vi "WVDIAL_2_OphirPM_v2.3_temp_tune.vi"() -> ()   [LabVIEW 2012]
uses:
  <vilib>/DAQmx/write.llb/DAQmx Write (Digital 1D Bool NChan 1Samp 1Line).vi
  <vilib>/DAQmx/miscellaneous.llb/DAQmx Fill In Error Info.vi
  under_development/AMCS_Data.vi
  <vilib>/Analysis/baseanly.llb/Mean (DBL).vi
  H2O_DIAL/LabVIEW-2012/Scalar_Data.vi
  H2O_DIAL/LabVIEW-2012/Bristol WM V2_31b/CLDevIFace.dll
  <vilib>/Analysis/NI_AALBase.lvlib
panel:
  out "error out 4":errorcluster
  out "error out 3":errorcluster
  out "error out 2":errorcluster
  out "error out":errorcluster
  out "AMCS_Profile":i32=208217
  out "FileHour":i32=17
  out "L_Count":i32=201042
  out "sigma_off_total":dbl[](array[numeric])=[5.545387503084242e-25, 5.506921512625635e-25, 5.468655063160739e-25, 5.430588031815433e-25, 5.39272028507623e-25, 5.35505167878492e-25, 5.317582058036299e-25, 5.280311257273803e-25, 5.243239100182651e-25, 5.206365399736143e-25, 5.169689958185842e-25, 5.133212567065494e-25, 5.096933007194568e-25, 5.060851048742239e-25, 5.024966451178001e-25, 4.989278963386338e-25, 4.953788323632695e-25, 4.918494259626275e-25, 4.883396488574925e-25, 4.848494717236001e-25, 4.813788641946174e-25, 4.779277948683017e-25, 4.744962313158126e-25, 4.710841400843162e-25, 4.676914867043271e-25, 4.643182356986159e-25, 4.609643505899978e-25, 4.576297939040525e-25, 4.543145271851358e-25, 4.510185109959037e-25, 4.477417049336712e-25, 4.444840676323304e-25, 4.412455567763804e-25, 4.3802612910682375e-25, 4.348257404317652e-25, 4.316443456338351e-25, 4.284818986840961e-25, 4.253383526463104e-25, 4.222136596891092e-25, 4.191077710978466e-25, 4.160206372783186e-25, 4.1295220777418144e-25, 4.09902431272516e-25, 4.0687125561240014e-25, 4.038586277999945e-25, 4.0086449401468787e-25, 3.978887996201128e-25, 3.9493148917382813e-25, 3.9199250643855913e-25, 3.890717943910424e-25, 3.8616929523256806e-25, 3.832849503983646e-25, 3.804187005685776e-25, 3.775704856767893e-25, 3.7474024492078913e-25, 3.7192791677202016e-25, 3.691334389844544e-25, 3.6635674860611747e-25, 3.6359778198783013e-25, 3.608564747899254e-25, 3.5813276199740633e-25, 3.5542657792324006e-25, 3.5273785622244977e-25, 3.5006652989779304e-25, 3.474125313105615e-25, 3.447757921904358e-25, 3.421562436422067e-25, 3.3955381615686624e-25, 3.3696843961848715e-25, 3.3440004331667853e-25, 3.318485559484839e-25, 3.2931390563522844e-25, 3.2679601992567473e-25, 3.2429482580501904e-25, 3.218102497081505e-25, 3.1934221752128248e-25, 3.1689065459536094e-25, 3.144554857534307e-25, 3.1203663529904646e-25, 3.096340270240214e-25, 3.072475842173334e-25, 3.0487722967580223e-25, 3.0252288570892426e-25, 3.0018447414936605e-25, 2.9786191636379327e-25, 2.955551332584365e-25, 2.93264045288151e-25, 2.9098857246799783e-25, 2.8872863437846284e-25, 2.8648415018058536e-25, 2.8425503861601494e-25, 2.8204121802703507e-25, 2.798426063570431e-25, 2.7765912116729236e-25, 2.7549067964110224e-25, 2.7333719859787194e-25, 2.711985945027861e-25, 2.6907478347596096e-25, 2.6696568130369055e-25, 2.6487120345168007e-25, 2.6279126507436266e-25, 2.607257810243747e-25, 2.586746658706325e-25, 2.566378339056027e-25, 2.5461519915940007e-25, 2.5260667541452756e-25, 2.506121762134075e-25, 2.486316148821428e-25, 2.4666490453505376e-25, 2.447119580936065e-25, 2.4277268830394e-25, 2.408470077462466e-25, 2.389348288547815e-25, 2.370360639362542e-25, 2.351506251801359e-25, 2.332784246834128e-25, 2.314193744632263e-25, 2.2957338648035625e-25, 2.2774037265327427e-25, 2.2592024487921483e-25, 2.2411291505941054e-25, 2.223182951101569e-25, 2.205362969947517e-25, 2.187668327386051e-25, 2.170098144538901e-25, 2.152651543607901e-25, 2.1353276481789486e-25, 2.118125583372691e-25, 2.1010444761621367e-25, 2.0840834556144e-25, 2.0672416530970137e-25, 2.0505182026574318e-25, 2.0339122412060197e-25, 2.0174229088077294e-25, 2.0010493489925423e-25, 1.984790709041639e-25, 1.9686461402712443e-25, 1.9526147983151476e-25, 1.9366958434601173e-25, 1.9208884409824196e-25, 1.9051917613704353e-25, 1.889604980701633e-25, 1.8741272810013844e-25, 1.8587578504559242e-25, 1.8434958838460569e-25, 1.8283405828232852e-25, 1.8132911562539594e-25, 1.7983468204941469e-25, 1.7835067998523628e-25, 1.7687703267884065e-25, 1.7541366422950964e-25, 1.7396049962212014e-25, 1.7251746476173548e-25, 1.7108448650539577e-25, 1.6966149269382962e-25, 1.682484121773569e-25, 1.6684517485976216e-25, 1.6545171171822567e-25, 1.6406795483257825e-25, 1.6269383742584355e-25, 1.6132929387733532e-25, 1.5997425976472618e-25, 1.5862867187545788e-25, 1.5729246824495738e-25, 1.559655881722198e-25, 1.5464797224504997e-25, 1.5333956236218115e-25, 1.5204030174906975e-25, 1.507501349795091e-25, 1.4946900799166377e-25, 1.4819686809608036e-25, 1.4693366399595516e-25, 1.4567934579476733e-25, 1.4443386500081363e-25, 1.4319717453365839e-25, 1.4196922873047534e-25, 1.4074998334857028e-25, 1.3953939555457824e-25, 1.383374239287782e-25, 1.3714402845348837e-25, 1.359591705025627e-25, 1.3478281283530872e-25, 1.3361491956400066e-25, 1.3245545615800712e-25, 1.3130438940239329e-25, 1.301616873745446e-25, 1.2902731942704976e-25, 1.279012561404225e-25, 1.267834693001398e-25, 1.2567393184886676e-25, 1.24572617844065e-25, 1.234795024159748e-25, 1.2239456171273316e-25, 1.2131777284818955e-25, 1.2024911384743837e-25, 1.1918856357986882e-25, 1.1813610169410398e-25, 1.1709170855643455e-25, 1.1605536517289937e-25, 1.150270531049662e-25, 1.140067544094941e-25, 1.1299445152854262e-25, 1.119901272247768e-25, 1.1099376447618997e-25, 1.100053463798013e-25, 1.0902485605823632e-25, 1.080522765581465e-25, 1.070875907298926e-25, 1.0613078113261455e-25, 1.0518182990591116e-25, 1.042407186678202e-25, 1.0330742837066907e-25, 1.0238193919447418e-25, 1.0146423040946438e-25, 1.0055428024548321e-25, 9.965206574741577e-26, 9.875756265476834e-26, 9.787074522931174e-26, 9.699158614073894e-26, 9.612005628632109e-26, 9.525612466180461e-26, 9.439975818936259e-26, 9.355092156100758e-26, 9.270957708501334e-26, 9.187568450780461e-26, 9.104920084865156e-26, 9.023008023764633e-26, 8.94182737331762e-26, 8.861372914237573e-26, 8.781639085901568e-26, 8.702619966455919e-26, 8.624309255898195e-26, 8.546700257831125e-26, 8.469785860384154e-26, 8.39355851772518e-26, 8.3180102322408e-26, 8.243132536126833e-26, 8.168916471875328e-26, 8.095352575467842e-26, 8.022430856855752e-26, 7.950140784015605e-26, 7.878471262861986e-26, 7.807410623725093e-26, 7.736946601808152e-26, 7.667066322910378e-26, 7.597756288463996e-26, 7.529002360167144e-26, 7.460789748985888e-26, 7.393103001654563e-26, 7.325925991061249e-26, 7.259241906883069e-26, 7.193033248448865e-26, 7.127281819541907e-26, 7.061968726910621e-26, 6.997074376832589e-26, 6.932578480231767e-26, 6.868460056400776e-26, 6.804697441376138e-26, 6.741268300427973e-26, 6.678149643381507e-26, 6.615317845700336e-26, 6.552748670734475e-26, 6.490417302477185e-26, 6.42829837718818e-26, 6.366366023790365e-26, 6.304593910876558e-26, 6.242955297230882e-26, 6.181423091318249e-26, 6.11996991406899e-26, 6.058568172515334e-26, 5.997190137859553e-26, 5.935808030604093e-26, 5.874394115193087e-26, 5.812920798981541e-26, 5.751360741508913e-26, 5.689686966977323e-26, 5.627872990055172e-26]
  out "sigma_on_total":dbl[](array[numeric])=[2.1897186319501164e-23, 2.1841487529678764e-23, 2.1784368378737784e-23, 2.1725842413801422e-23, 2.1665923609093122e-23, 2.1604626360114625e-23, 2.1541965469976876e-23, 2.147795614304285e-23, 2.1412613971127952e-23, 2.1345954924526415e-23, 2.1277995341118866e-23, 2.120875191483118e-23, 2.113824168388313e-23, 2.106648202099629e-23, 2.099349061869916e-23, 2.0919285481354415e-23, 2.0843884909288052e-23, 2.0767307489252352e-23, 2.0689572080890114e-23, 2.061069780525927e-23, 2.0530704031971798e-23, 2.0449610366258792e-23, 2.036743663641153e-23, 2.0284202882924402e-23, 2.019992934281886e-23, 2.0114636440052182e-23, 2.00283447706975e-23, 1.9941075090753357e-23, 1.985284830485466e-23, 1.976368545197079e-23, 1.9673607693776973e-23, 1.958263630178374e-23, 1.9490792645419655e-23, 1.9398098179769622e-23, 1.9304574432981866e-23, 1.9210242993792915e-23, 1.911512550178836e-23, 1.9019243632147982e-23, 1.892261908749492e-23, 1.882527358382039e-23, 1.8727228840484137e-23, 1.862850656865659e-23, 1.8529128460810584e-23, 1.842911617911315e-23, 1.8328491345744676e-23, 1.8227275532131632e-23, 1.8125490248401552e-23, 1.8023156934769116e-23, 1.792029694973319e-23, 1.78169315636254e-23, 1.771308194643307e-23, 1.76087691601277e-23, 1.7504014150381522e-23, 1.7398837737268475e-23, 1.7293260607489634e-23, 1.718730330643124e-23, 1.7080986230482727e-23, 1.6974329619201828e-23, 1.6867353548578025e-23, 1.6760077923728236e-23, 1.665252247268762e-23, 1.654470674045623e-23, 1.6436650081676406e-23, 1.6328371654819108e-23, 1.6219890418650818e-23, 1.6111225124499464e-23, 1.6002394312440044e-23, 1.5893416306119294e-23, 1.5784309208642462e-23, 1.567509089831123e-23, 1.5565779023438924e-23, 1.5456391000184535e-23, 1.534694400825861e-23, 1.523745498728377e-23, 1.5127940634948223e-23, 1.501841740268206e-23, 1.490890149504341e-23, 1.479940886472835e-23, 1.4689955213544446e-23, 1.4580555988261152e-23, 1.447122637936001e-23, 1.4361981321097285e-23, 1.4252835487670488e-23, 1.414380329480521e-23, 1.4034898897080252e-23, 1.3926136188406203e-23, 1.3817528800853457e-23, 1.3709090104403687e-23, 1.3600833207945943e-23, 1.349277095793143e-23, 1.3384915938652766e-23, 1.3277280474775945e-23, 1.3169876628752232e-23, 1.3062716204007209e-23, 1.2955810745104247e-23, 1.2849171537735469e-23, 1.2742809611585541e-23, 1.2636735740242556e-23, 1.2530960443282978e-23, 1.2425493987127416e-23, 1.2320346388003672e-23, 1.2215527411383842e-23, 1.2111046577113862e-23, 1.2006913157446616e-23, 1.1903136182976424e-23, 1.1799724441226872e-23, 1.169668648174857e-23, 1.1594030616501561e-23, 1.1491764922867505e-23, 1.1389897246703087e-23, 1.1288435203607327e-23, 1.1187386182417802e-23, 1.1086757346926609e-23, 1.0986555640361757e-23, 1.0886787785418347e-23, 1.0787460289424461e-23, 1.0688579445960512e-23, 1.0590151337721473e-23, 1.0492181840266546e-23, 1.0394676623216386e-23, 1.0297641155480216e-23, 1.0201080705953425e-23, 1.0105000348200365e-23, 1.000940496261448e-23, 9.914299238906325e-24, 9.819687681041688e-24, 9.725574608371918e-24, 9.631964159237653e-24, 9.538860294547854e-24, 9.446266800038345e-24, 9.354187289596407e-24, 9.262625209327728e-24, 9.171583838293643e-24, 9.081066293599967e-24, 8.991075533143189e-24, 8.901614357381249e-24, 8.812685413580547e-24, 8.724291198059886e-24, 8.636434059883374e-24, 8.549116202846888e-24, 8.46233968936254e-24, 8.376106442190555e-24, 8.290418248957488e-24, 8.205276763614756e-24, 8.120683509296393e-24, 8.036639882480817e-24, 7.953147154190918e-24, 7.870206473431928e-24, 7.787818870345368e-24, 7.705985257815232e-24, 7.624706435006336e-24, 7.543983089983992e-24, 7.463815801475284e-24, 7.384205042284291e-24, 7.305151181813397e-24, 7.226654487950019e-24, 7.148715130145818e-24, 7.071333180855378e-24, 6.994508619523118e-24, 6.918241333557414e-24, 6.842531121444102e-24, 6.767377694272425e-24, 6.692780678760056e-24, 6.618739619458455e-24, 6.5452539800133945e-24, 6.472323146426738e-24, 6.3999464282545864e-24, 6.328123061586831e-24, 6.256852210192852e-24, 6.1861329678933266e-24, 6.1159643610427095e-24, 6.046345349428136e-24, 5.977274829030023e-24, 5.908751633539751e-24, 5.8407745358644116e-24, 5.773342250582962e-24, 5.7064534355285664e-24, 5.6401066928767316e-24, 5.574300571639491e-24, 5.509033568997274e-24, 5.444304131618612e-24, 5.380110657866868e-24, 5.31645149889479e-24, 5.2533249603231364e-24, 5.190729303587478e-24, 5.128662747548667e-24, 5.0671234700616424e-24, 5.00610960894438e-24, 4.9456192636359835e-24, 4.885650496667281e-24, 4.826201334553736e-24, 4.767269769352692e-24, 4.708853759908912e-24, 4.650951232941731e-24, 4.5935600842415034e-24, 4.536678180090787e-24, 4.480303358139369e-24, 4.42443342839447e-24, 4.36906617468056e-24, 4.314199355323438e-24, 4.259830704429773e-24, 4.2059579327711866e-24, 4.1525787289997016e-24, 4.0996907601349414e-24, 4.047291672739682e-24, 3.995379094165581e-24, 3.943950632649501e-24, 3.893003879184515e-24, 3.842536407255649e-24, 3.7925457746476135e-24, 3.743029523589732e-24, 3.693985181959847e-24, 3.645410263417867e-24, 3.597302269072591e-24, 3.549658687175159e-24, 3.502476994826442e-24, 3.455754657754984e-24, 3.409489131383154e-24, 3.363677861749587e-24, 3.318318285465553e-24, 3.273407830893777e-24, 3.2289439184542047e-24, 3.1849239612908476e-24, 3.1413453657394826e-24, 3.0982055320457536e-24, 3.0555018547123555e-24, 3.013231722929312e-24, 2.9713925214102524e-24, 2.929981630614343e-24, 2.8889964270553894e-24, 2.848434284325051e-24, 2.808292572802531e-24, 2.768568660723256e-24, 2.729259914040449e-24, 2.6903636973694872e-24, 2.6518773738399542e-24, 2.613798305854699e-24, 2.5761238554459867e-24, 2.5388513841964624e-24, 2.5019782541616026e-24, 2.4655018278391552e-24, 2.4294194684970563e-24, 2.393728540690758e-24, 2.3584264104242274e-24, 2.3235104453130033e-24, 2.288978015131802e-24, 2.2548264920156124e-24, 2.221053250472187e-24, 2.1876556679564417e-24, 2.154631124988252e-24, 2.121977005391232e-24, 2.0896906964654865e-24, 2.0577695892720847e-24, 2.0262110789046935e-24, 1.9950125645818837e-24, 1.9641714498520942e-24, 1.9336851429527643e-24, 1.903551056829774e-24, 1.873766609217632e-24, 1.8443292231846464e-24, 1.8152363269306076e-24, 1.7864853541592603e-24, 1.758073744034404e-24, 1.7299989416783995e-24, 1.7022583979224166e-24, 1.674849569693973e-24, 1.6477699200554648e-24, 1.6210169183820797e-24, 1.5945880404417097e-24, 1.568480768561727e-24, 1.5426925917440813e-24, 1.5172210056495893e-24, 1.492063512922192e-24, 1.4672176231213581e-24, 1.4426808528675062e-24, 1.4184507260582342e-24, 1.3945247736815164e-24]
  out "background start":u32=254
  in  "Tab Control 2":enum32{"WV ND Narrow", "WV ND Wide"}(tab)
  out "Water Vapor Number Density":dbl[][](graph)=[[1.1686220819599875, 1.4774367217267463, 1.9038758293418794, 1.8830179059073306, 2.0440576087457822, 2.1668624597271653, 1.97937019383078, 1.5621924545527897, 1.1664740318450977, 2.0754647898565035, 2.747080898464423, 1.8916405098017475, 1.0874207989422877, 0.93835383425456, 1.6290167760793863, 2.0629058736674017, 1.4999472708715333, 1.672997855512388, 1.6553848412331555, 1.3148311142843476, 1.6421554693618547, 1.370698833697994, 1.20191305319464, 0.8655598598379174, 0.5658145450310454, 1.4737101750069286, 2.1438967428140137, 1.5774205481436212, 0.08010163904850712, 0.4966991501349844, 1.7922589218677836, -0.45393082568851406, -1.640669951809988, 1.4950245551019732, 2.877460933764352, 2.481262841347946, 1.2612337541825702, -1.313721337625759, -1.46621373625896, 1.4661798903302752, 1.3081549860140265, 1.156849905625117, 0.8714019244452782, 1.577440623355066, 1.9842036647458816, 0.29054369655614604, 0.12181866131521751, 1.1799250362012412, 0.44848635334858383, -0.05394343532656153, -0.2493439710627751, 0.8995169233937147, 0.692659116354861, -0.8664603283818014, -1.188125394340996, 0.009767610923537213, 0.05408639955157989, -0.43086138298632376, 0.2378520561582474, 0.945019145078991, 0.8770759959531872, -4.740703995285504, -10.205482356490268, -5.843085236768064, 8.32319036475107, -4.931763620409371, -4.640820493623135, -2.6493628781520115, -4.983100868146263, -9.024714982302626, -8.561689566051607, -1.830756894538194, -10.987315517233569, -16.304802271628947, -11.589931756630762, -8.465109314093807, -3.068957925785124, -1.4086959240175307, 2.6119539574875628, -1.1232277890861027, -0.0010841988213187153, -6.786838123899488, 19.784020463078896, 12.58471640147054, -3.2017264576194195, 20.717734726764544, 12.988472818052779, 8.300076780687139, 5.5609290756076355, 12.35871399176313, 10.323554724189568, 14.452942516815366, 3.258642961310386, 13.138932169359636, 10.053800283197544, -3.791863029393354, -2.7086939678120037, -1.2343342544259563, 3.3604040363855736, 1.2847662491408278, 1.1614512114400366, 4.707724407239739, 6.483551952142477, 0.35714346017500526, -4.090275309901479, -3.877615477608852, -2.0316244199809432, -10.062704071811757, -14.143459495969896, -14.063233569103849, -18.553158750204265, -13.983874134364614, -12.455424626276272, 8.556352909957788, -4.660280260049854, 8.076420102443958, -15.996110767990778, -4.554140066978605, 9.41403379044399, 0.49053083794270463, -1.9489101364871924, -1.3796083872589544, -0.8630424656038397, -8.749400736117634, -10.240997395328117, -27.49373961788248, 23.711146628275404, 11.747115184638806, -16.313121770166735, -20.12049027647351, 2.4764954440857667, 3.118314957311149, -3.4978447490739084, -7.490695667548567, 6.94536111281849, -0.5770115269917374, 6.837627961343941, -12.798595899669873, -7.552034774653854, 9.613345509180892, -5.834038094450012, -5.244620526296466, -0.33499029121524715, -19.19675593892565, -21.858436759386162, 1.6653621297819792, 5.200681478690842, 17.088876238099946, -26.399330226594188, -30.94010982572226, -18.95654187193061, -1.3410548888034564, 33.35879499985644, 9.171534190818264, -16.26525455458909, 23.977605764747285, -29.83483396783575, 8.029426001754773, 26.078663692822328, 40.82483770932593, 34.742116444245234, 6.566292022612825, -34.92666994493613, 13.553331396566898, 22.437200410977113, -19.37495162442004, 34.4712113783406, -46.69604527818464, 62.765870932862086, 14.03770220887764, -5.2864336092955835, -8.043212616718813, -15.494425006820387, -14.848350127425917, 0.06803737836791812, -3.3667429378906233, 33.72917397268682, 41.14798130944211, -52.357973020530736, -5.66115980307453, -4.772944453482474, 10.197774334791216, 14.301342615722469, 2.7869855224906845, 15.547682901084972, 24.461354106351042, -54.35802691769603, -18.692953443590284, 0.5819768370065017, -22.710229897699826, 53.510038445268826, 17.171252849821453, -67.38074518593801, -9.275668760548527, -39.79303339707957, -16.616815117683064, 65.0884708353045, 8.11037403035155, 27.670242971359876, -45.54768779130534, -75.97133775948198, -43.04948657067137, 45.66148580215234, -26.551912052229547, 18.458130931307903, -17.37228096859303, -89.97450123677359, -29.325724485113035, 25.301892410855, 66.34159930996725, -30.347348250261653, -50.559785062063234, 7.689890863200726, 88.04583527549127, 3.9623539367017595, -66.72419744097765, 18.617576881641398, 51.80174756239796, -138.3410501919035, -44.87865875264082, 79.64184742294394, -120.93925552570147, 19.824468913556238, 66.24303807213145, -11.84147299236148, -8.469978895050494, -42.84267466311351, -24.93121030553229, 126.4282227857208, 31.046670771709834, -35.415078757055696, 157.35776829630527, -35.33392033521813, -102.69456860831939, 51.53770911950967, 184.21868875607393, 52.399040902191246, 47.78246920683896, -27.75521755383029, 30.781302029149078, 69.20085683283433, -9.814996999502586, 33.2921680158996, -50.39721028467972, -16.175857426206594, 37.52360534064173, -9.996678873705923, -10.305741295302573, -16.626421650465023, 30.847714338931155, 81.34545035962368, 92.0934893629275, 5.547876454714627, -121.63695316868021, -33.88737209024075, -156.47676665854917, -38.59121686147064, -37.11469155973703, -20.696842681631523, -3.6982168426823345, -134.68419720598982, -10.555438560814542, -46.88331213576928, 38.95833328472374, 55.217515895913756, -6.63079174875619, -18.762609922967414, -108.98184047128015, -4.8076844288237135, -29.06788122254778, -48.79027665089365, -84.51647284455252, -7.440719627565783, 74.0807845886109, -74.48676761809652, -11.866125520153098, 0.0, 0.0, 0.0, 0.0]]
  out "Water Vapor Number Density 2":dbl[][](graph)=[[nan, nan, nan, nan, nan, nan, nan, nan, nan, nan, nan, nan, nan, nan, nan, nan, nan, nan, nan, nan, nan, nan, nan, nan, nan, nan, nan, nan, nan, nan, nan, nan, nan, nan, nan, nan, nan, nan, nan, nan, nan, nan, nan, nan, nan, nan, nan, nan, nan, nan, nan, nan, nan, nan, nan, nan, nan, nan, nan, nan, nan, nan, nan, nan, nan, nan, nan, nan, nan, nan, nan, nan, nan, nan, nan, nan, nan, nan, nan, nan, nan, nan, nan, nan, nan, nan, nan, nan, nan, nan, nan, nan, nan, nan, nan, nan, nan, nan, nan, nan, nan, nan, nan, nan, nan, nan, nan, nan, nan, nan, nan, nan, nan, nan, nan, nan, nan, nan, nan, nan, nan, nan, nan, nan, nan, nan, nan, nan, nan, nan, nan, nan, nan, nan, nan, nan, nan, nan, nan, nan, nan, nan, nan, nan, nan, nan, nan, nan, nan, nan, nan, nan, nan, nan, nan, nan, nan, nan, nan, nan, nan, nan, nan, nan, nan, nan, nan, nan, nan, nan, nan, nan, nan, nan, nan, nan, nan, nan, nan, nan, nan, nan, nan, nan, nan, nan, nan, nan, nan, nan, nan, nan, nan, nan, nan, nan, nan, nan, nan, nan, nan, nan, nan, nan, nan, nan, nan, nan, nan, nan, nan, nan, nan, nan, nan, nan, nan, nan, nan, nan, nan, nan, nan, nan, nan, nan, nan, nan, nan, nan, nan, nan, nan, nan, nan, nan, nan, nan, nan, nan, nan, nan, nan, nan, nan, nan, nan, nan, nan, nan, nan, nan, nan, nan, nan, nan, nan, nan, nan, nan, nan, nan, nan, nan, nan, nan, nan, nan, nan, nan, nan, nan, nan, nan, nan, nan, 0.0, 0.0, 0.0, 0.0]] caption="Water Vapor Number Density"
  out "RingBuffer offline near":dbl[][](array[numeric])
  out "RingBuffer aerosol near":dbl[][](array[numeric])
  in  "LOWER DISPLAY TAB":T1(tab)=enum."Raw Counts Narrow"
  out "NRB":dbl[][](graph)=[[6.655721295710694e-05, 0.00037202741947904344, 0.0010501837810888938, 0.002260818770771549, 0.004166049017417403, 0.006889205383898037, 0.011051685681266066, 0.016620791809273314, 0.02497452746588639, 0.03551848686428863, 0.04598337939829831, 0.060078647321129525, 0.07935699801467896, 0.1005610372369731, 0.12257229368961048, 0.15078191065236987, 0.18372787433526802, 0.21495802589058974, 0.2511435905284201, 0.28417262954243927, 0.30641231672750574, 0.3366211082587094, 0.3587410049770007, 0.33324534901972924, 0.28122146881455035, 0.24457853857932904, 0.23311510592107937, 0.22090379799738227, 0.2071168499314668, 0.21382586314521793, 0.23577821239004024, 0.26304334168077026, 0.282359461516476, 0.2967104747137421, 0.2934990876387134, 0.2796972895140803, 0.28047679283540755, 0.2705144727293366, 0.2519952392940683, 0.2514362116457461, 0.26286175461298344, 0.25372471452451223, 0.25123251111722794, 0.2556233856397539, 0.24842534751068593, 0.24750981894971588, 0.25763651272890137, 0.28478695517617364, 0.2797118644363096, 0.258406264468613, 0.2642745252675272, 0.2738711346241327, 0.2816393893275038, 0.2676815908453075, 0.2534533185771932, 0.24539387779665767, 0.2622158317229759, 0.28033145866553966, 0.29350136280117894, 26.89391905102691, 117.07164418260645, 228.13032383043225, 202.51026324159363, 83.90785874658836, 15.757743022488503, 0.4234112909858623, -0.024984691370996244, -0.04685268874992606, -0.034764385663156226, -0.05112868567698688, -0.04327760916930205, -0.03482044006279036, -0.030162757086217157, -0.0062958751636364345, -0.03640264266141257, -0.07803494737427145, -0.02673358081237267, 0.018840384311627344, -0.019895836655699124, -0.06134567697619042, -0.06499364842870389, -0.02828790463804423, -0.04549274511785383, -0.06963084914012556, -0.03993991563497018, -0.0350231103042986, -0.07226518797771685, -0.03652489204584916, 0.04067498109234416, 0.026917864341533423, 0.03470885324679451, 0.09027180290224025, 0.06596158715982604, 0.11175180571495605, 0.17547278258513402, 0.17135750843049274, 0.15700690748958193, 0.09155363947186952, 0.09287662798984249, 0.13307990109336063, 0.0325521861948075, 0.000604765884959244, 0.013831413373720276, -0.024682796140254676, 0.01978376550606942, -0.014614681057396257, -0.056808466058083984, 0.040082576565457745, 0.07670703234848908, -0.011399697156017337, -0.013235606247373266, 0.018721602841350927, -0.03082651996114866, -0.06522024511701581, -0.004722281270442021, 0.029225240552739614, -0.01961371625467179, -0.06803802715765754, 2.1380604131926046e-05, 0.0924268129152713, 0.09010492757502066, -0.012898972695371968, -0.05108525018653476, -0.0005571608008071935, 0.010639581815176597, 0.0416724782939333, 0.06608075814228832, 0.10114108802800284, 0.07979940595584598, -0.051324427203699556, -0.22083876738177594, -0.14399754622889738, 0.04709907713140535, -0.005056076937183718, -0.14167534100413592, -0.09142572571769413, -0.04672837980028117, -0.15702637349931287, -0.14363241180128106, -0.08504650773624196, -0.04461930207647395, 0.10582724603656488, 0.07837656702649838, 0.03368743478950975, -0.14519059414991406, -0.20311272007260686, -0.03259281671207828, -0.13431311346920413, -0.15079785748764288, -0.047100168125256324, -0.026214800877661495, -0.01697047379964134, 0.05260949901048305, 0.06896552982000768, 0.17597121786673345, 0.09878633626569339, -0.04043434336110266, -0.20489726628957777, -0.14643299654359876, 0.1628647821117614, 0.24318730528379853, 0.11990520883496149, -0.05611938909287257, -0.18725613924310366, 0.11308275739412733, 0.16906745383528887, -0.22522080967176134, -0.12779331611685849, -0.16650943190315967, -0.09540341909442, 0.00611460823616924, -0.2774294997534905, -0.09767067044269935, 0.17204129185178976, -0.0016876984432913778, -0.17532774695114706, -0.13121004078584492, -0.1769434242045843, -0.17470452352862337, 0.03368045654278133, 0.0019043382503988726, -0.26624649905849934, -0.3646050922321933, -0.23187986598476729, -0.45011643572206855, -0.22846088112894056, -0.07254209020362341, -0.18471031559246315, -0.1340995723684058, -0.1729921834231155, -0.037123573059500176, -0.020120336755339932, 0.1237856208466393, 0.1321749783814788, 0.04455129540045739, 0.03413400073974604, -0.0409574263170348, -0.05173257415190935, -0.16510694259121034, -0.2543341498601033, -0.24925968300475004, -0.21478473705848852, -0.16403424557507149, -0.12010260802481695, -0.10066233524155897, -0.15930823473658823, -0.1948213799148583, -0.07586944721918257, -0.2324017094755593, -0.33366507802042705, -0.304924489411266, -0.2696550078446261, -0.136927104518987, -0.2436544192473321, -0.28780864509755266, -0.30634034569121554, -0.4362543647415865, -0.34253176865566803, 0.002787887025041371, -0.0510793742107368, -0.15017105217208448, 0.021467380603209536, 0.050755765605681104, 0.0635226731289704, -0.0562938117166624, -0.03655267970882738, 0.3638081558134828, 0.23162086386658876, -0.34927239870794163, -0.4870954199260063, -0.4732151203964187, -0.3615307418865022, -0.12901369884584193, -0.05262031250017241, -0.23545845082907382, -0.3835641923235008, -0.08683969260532591, 0.07064209484407737, 0.05075406747852546, -0.08796502961716723, 0.011049209779137618, 0.2653601576936556, -0.026656829322920347, -0.032494693171276005, -0.17209766914365482, -0.5709260148556188, -0.35222594464206175, -0.4665061455314845, -0.1602117120020841, 0.17113208614366154, -0.018928914364878476, -0.27555068506542396, -0.06634446073711907, 0.31546512043081887, -0.20852194047387598, -0.4525665055033898, 0.1696305000463501, 0.24381853506510856, -0.14168936503966975, 0.012860084727702744, 0.18652302144307786, 0.41986371481437895, 0.9466132410659908, 0.7222859069991262, 0.3221737406060694, 0.07622305891934592, -0.1694129119530885, -0.19237188369018504, -0.5242768208612977, -0.3410843427529666, -0.14680704658065782, -0.19676094672880415, -0.5202944838977543, -0.4575248827370781, -0.37096004141438943, -0.21840419899520275, 0.20140385405739533, 0.0, 0.0, 0.0]] caption="Water Vapor Number Density"
  out "NRB 2":dbl[][](graph) caption="Water Vapor Number Density"
  out "raw counts":dbl[][](graph)=[[27.799999999999955, 103.79999999999995, 56.799999999999955, 88.79999999999995, 178.79999999999995, 168.79999999999995, 198.79999999999995, 241.79999999999995, 291.79999999999995, 316.79999999999995, 380.79999999999995, 352.79999999999995, 437.79999999999995, 431.79999999999995, 578.8, 436.79999999999995, 549.8, 536.8, 604.8, 671.8, 613.8, 643.8, 592.8, 577.8, 470.79999999999995, 351.79999999999995, 316.79999999999995, 323.79999999999995, 251.79999999999995, 184.79999999999995, 237.79999999999995, 233.79999999999995, 231.79999999999995, 244.79999999999995, 271.79999999999995, 168.79999999999995, 178.79999999999995, 158.79999999999995, 69.79999999999995, 146.79999999999995, 90.79999999999995, 153.79999999999995, 76.79999999999995, 162.79999999999995, 103.79999999999995, 101.79999999999995, 118.79999999999995, 96.79999999999995, 100.79999999999995, 63.799999999999955, 117.79999999999995, 84.79999999999995, 95.79999999999995, 81.79999999999995, 107.79999999999995, 37.799999999999955, 62.799999999999955, 100.79999999999995, 66.79999999999995, 69.79999999999995, 14790.8, 43026.8, 40243.8, 11146.8, 613.8, 20.799999999999955, -22.200000000000045, -67.20000000000005, 33.799999999999955, -60.200000000000045, -4.2000000000000455, 1.7999999999999545, 15.799999999999955, -27.200000000000045, -9.200000000000045, -18.200000000000045, -4.2000000000000455, 19.799999999999955, 18.799999999999955, -2.2000000000000455, -8.200000000000045, 37.799999999999955, -46.200000000000045, 47.799999999999955, 10.799999999999955, 17.799999999999955, -18.200000000000045, -39.200000000000045, -1.2000000000000455, 0.7999999999999545, 16.799999999999955, 5.7999999999999545, 20.799999999999955, -45.200000000000045, 19.799999999999955, 13.799999999999955, -23.200000000000045, -19.200000000000045, 59.799999999999955, 5.7999999999999545, -16.200000000000045, 26.799999999999955, 56.799999999999955, 0.7999999999999545, -1.2000000000000455, -34.200000000000045, 28.799999999999955, -55.200000000000045, -7.2000000000000455, -1.2000000000000455, -7.2000000000000455, 7.7999999999999545, -10.200000000000045, 8.799999999999955, 16.799999999999955, 23.799999999999955, -29.200000000000045, 2.7999999999999545, -4.2000000000000455, 9.799999999999955, 55.799999999999955, 20.799999999999955, -23.200000000000045, 4.7999999999999545, -72.20000000000005, -25.200000000000045, -10.200000000000045, 55.799999999999955, 14.799999999999955, -5.2000000000000455, 3.7999999999999545, 14.799999999999955, -25.200000000000045, 63.799999999999955, 4.7999999999999545, -45.200000000000045, -8.200000000000045, -55.200000000000045, -31.200000000000045, 13.799999999999955, 17.799999999999955, 22.799999999999955, -25.200000000000045, 43.799999999999955, 20.799999999999955, 0.7999999999999545, 26.799999999999955, -13.200000000000045, -7.2000000000000455, -35.200000000000045, 15.799999999999955, 3.7999999999999545, 9.799999999999955, 41.799999999999955, -2.2000000000000455, 16.799999999999955, 14.799999999999955, -46.200000000000045, 19.799999999999955, 1.7999999999999545, 22.799999999999955, 7.7999999999999545, -32.200000000000045, 20.799999999999955, -14.200000000000045, -15.200000000000045, -3.2000000000000455, -8.200000000000045, 11.799999999999955, -20.200000000000045, 22.799999999999955, 42.799999999999955, 2.7999999999999545, -35.200000000000045, 47.799999999999955, 28.799999999999955, -24.200000000000045, 10.799999999999955, 20.799999999999955, -7.2000000000000455, 9.799999999999955, -11.200000000000045, -10.200000000000045, -50.200000000000045, -32.200000000000045, -2.2000000000000455, 0.7999999999999545, -66.20000000000005, 1.7999999999999545, 4.7999999999999545, -17.200000000000045, -40.200000000000045, 12.799999999999955, 44.799999999999955, 33.799999999999955, -5.2000000000000455, -20.200000000000045, 8.799999999999955, -25.200000000000045, -33.200000000000045, -60.200000000000045, -2.2000000000000455, -73.20000000000005, -0.20000000000004547, 43.799999999999955, -15.200000000000045, 14.799999999999955, 5.7999999999999545, -28.200000000000045, -29.200000000000045, -19.200000000000045, -24.200000000000045, -12.200000000000045, 23.799999999999955, -3.2000000000000455, 6.7999999999999545, 15.799999999999955, -32.200000000000045, 5.7999999999999545, 6.7999999999999545, -68.20000000000005, -1.2000000000000455, -36.200000000000045, 10.799999999999955, -40.200000000000045, -8.200000000000045, 24.799999999999955, 50.799999999999955, 42.799999999999955, 2.7999999999999545, 5.7999999999999545, -20.200000000000045, -28.200000000000045, 36.799999999999955, 6.7999999999999545, -29.200000000000045, 24.799999999999955, 20.799999999999955, -6.2000000000000455, -2.2000000000000455, 31.799999999999955, 17.799999999999955, -5.2000000000000455, 92.79999999999995, -0.20000000000004547, -2.2000000000000455, -84.20000000000005, 2.7999999999999545, -15.200000000000045, -22.200000000000045, -30.200000000000045, 7.7999999999999545, 0.7999999999999545, 23.799999999999955, 35.799999999999955, 0.7999999999999545, -37.200000000000045, 2.7999999999999545, 20.799999999999955, -38.200000000000045, 19.799999999999955, -39.200000000000045, -47.200000000000045, 27.799999999999955, -72.20000000000005, 33.799999999999955, 35.799999999999955, -3.2000000000000455, -30.200000000000045, -17.200000000000045, 31.799999999999955, -19.200000000000045, -29.200000000000045, 41.799999999999955, 15.799999999999955, -2.2000000000000455, 10.799999999999955, 5.7999999999999545, 51.799999999999955, 0.0]] caption="Water Vapor Number Density"
  out "raw counts near":dbl[][](graph) caption="Water Vapor Number Density"
  out "Aerosol Smoothed 2":dbl[](array[numeric])
  out "Off-Line Smoothed 2":dbl[](array[numeric])
  out "Off-Line Bin Readings 2":dbl[](array[numeric])
  out "On-Line Smoothed 2":dbl[](array[numeric])
  out "On-Line Bin Readings 2":dbl[](array[numeric])
  in  "stop":bool
  in  "Reset Average":bool=TRUE
  in  "Save Data?":bool=TRUE
  in  "Collect Data?":bool=TRUE
  in  "Tab Control":T2(tab)=enum."OD"
  out "Water Vapor Number Density  2":cluster{"Y":dbl[], "Y":dbl[]}[](graph)=[{"Y"=array[276 elements], "Y"=array[280 elements]}, {"Y"=[nan, nan, nan, nan, nan, nan, nan, nan, nan, nan, nan, nan, nan, nan, nan, nan, nan, nan, nan, nan, nan, nan, nan, nan, nan, nan, nan, nan, nan, nan, nan, nan, nan, nan, nan, nan, nan, nan, nan, nan, nan, nan, nan, nan, nan, nan, nan, nan, nan, nan, nan, nan, nan, nan, nan, nan, nan, nan, nan, nan, nan, nan, nan, nan, nan, nan, nan, nan, nan, nan, nan, nan, nan, nan, nan, nan, nan, nan, nan, nan, nan, nan, nan, nan, nan, nan, nan, nan, nan, nan, nan, nan, nan, nan, nan, nan, nan, nan, nan, nan, nan, nan, nan, nan, nan, nan, nan, nan, nan, nan, nan, nan, nan, nan, nan, nan, nan, nan, nan, nan, nan, nan, nan, nan, nan, nan, nan, nan, nan, nan, nan, nan, nan, nan, nan, nan, nan, nan, nan, nan, nan, nan, nan, nan, nan, nan, nan, nan, nan, nan, nan, nan, nan, nan, nan, nan, nan, nan, nan, nan, nan, nan, nan, nan, nan, nan, nan, nan, nan, nan, nan, nan, nan, nan, nan, nan, nan, nan, nan, nan, nan, nan, nan, nan, nan, nan, nan, nan, nan, nan, nan, nan, nan, nan, nan, nan, nan, nan, nan, nan, nan, nan, nan, nan, nan, nan, nan, nan, nan, nan, nan, nan, nan, nan, nan, nan, nan, nan, nan, nan, nan, nan, nan, nan, nan, nan, nan, nan, nan, nan, nan, nan, nan, nan, nan, nan, nan, nan, nan, nan, nan, nan, nan, nan, nan, nan, nan, nan, nan, nan, nan, nan, nan, nan, nan, nan, nan, nan, nan, nan, nan, nan, nan, nan, nan, nan, nan, nan, nan, nan, nan, nan, nan, nan, nan, nan], "Y"=array[280 elements]}]
  out "Absolute Humidity":cluster{"Y":dbl[], "Y":dbl[]}[](graph)=[{"Y"=array[276 elements], "Y"=array[280 elements]}, {"Y"=[nan, nan, nan, nan, nan, nan, nan, nan, nan, nan, nan, nan, nan, nan, nan, nan, nan, nan, nan, nan, nan, nan, nan, nan, nan, nan, nan, nan, nan, nan, nan, nan, nan, nan, nan, nan, nan, nan, nan, nan, nan, nan, nan, nan, nan, nan, nan, nan, nan, nan, nan, nan, nan, nan, nan, nan, nan, nan, nan, nan, nan, nan, nan, nan, nan, nan, nan, nan, nan, nan, nan, nan, nan, nan, nan, nan, nan, nan, nan, nan, nan, nan, nan, nan, nan, nan, nan, nan, nan, nan, nan, nan, nan, nan, nan, nan, nan, nan, nan, nan, nan, nan, nan, nan, nan, nan, nan, nan, nan, nan, nan, nan, nan, nan, nan, nan, nan, nan, nan, nan, nan, nan, nan, nan, nan, nan, nan, nan, nan, nan, nan, nan, nan, nan, nan, nan, nan, nan, nan, nan, nan, nan, nan, nan, nan, nan, nan, nan, nan, nan, nan, nan, nan, nan, nan, nan, nan, nan, nan, nan, nan, nan, nan, nan, nan, nan, nan, nan, nan, nan, nan, nan, nan, nan, nan, nan, nan, nan, nan, nan, nan, nan, nan, nan, nan, nan, nan, nan, nan, nan, nan, nan, nan, nan, nan, nan, nan, nan, nan, nan, nan, nan, nan, nan, nan, nan, nan, nan, nan, nan, nan, nan, nan, nan, nan, nan, nan, nan, nan, nan, nan, nan, nan, nan, nan, nan, nan, nan, nan, nan, nan, nan, nan, nan, nan, nan, nan, nan, nan, nan, nan, nan, nan, nan, nan, nan, nan, nan, nan, nan, nan, nan, nan, nan, nan, nan, nan, nan, nan, nan, nan, nan, nan, nan, nan, nan, nan, nan, nan, nan, nan, nan, nan, nan, nan, nan], "Y"=array[280 elements]}]
  out "NRB plot":cluster{"Y":dbl[], "Y":dbl[]}[](graph)
  in  "background length":i32=25
  out "Correction":cluster{"Y":dbl[], "Y":dbl[]}[](graph)=[{"Y"=array[277 elements], "Y"=array[280 elements]}, {"Y"=[1.0, 1.0, 1.0, 1.0, 1.0, 1.0, 1.0, 1.0, 1.0, 1.0, 1.0, 1.0, 1.0, 1.0, 1.0, 1.0, 1.0, 1.0, 1.0, 1.0, 1.0, 1.0, 1.0, 1.0, 1.0, 1.0, 1.0, 1.0, 1.0, 1.0, 1.0, 1.0, 1.0, 1.0, 1.0, 1.0, 1.0, 1.0, 1.0, 1.0, 1.0, 1.0, 1.0, 1.0, 1.0, 1.0, 1.0, 1.0, 1.0, 1.0, 1.0, 1.0, 1.0, 1.0, 1.0, 1.0, 1.0, 1.0, 1.0, 1.0, 1.0, 1.0, 1.0, 1.0, 1.0, 1.0, 1.0, 1.0, 1.0, 1.0, 1.0, 1.0, 1.0, 1.0, 1.0, 1.0, 1.0, 1.0, 1.0, 1.0, 1.0, 1.0, 1.0, 1.0, 1.0, 1.0, 1.0, 1.0, 1.0, 1.0, 1.0, 1.0, 1.0, 1.0, 1.0, 1.0, 1.0, 1.0, 1.0, 1.0, 1.0, 1.0, 1.0, 1.0, 1.0, 1.0, 1.0, 1.0, 1.0, 1.0, 1.0, 1.0, 1.0, 1.0, 1.0, 1.0, 1.0, 1.0, 1.0, 1.0, 1.0, 1.0, 1.0, 1.0, 1.0, 1.0, 1.0, 1.0, 1.0, 1.0, 1.0, 1.0, 1.0, 1.0, 1.0, 1.0, 1.0, 1.0, 1.0, 1.0, 1.0, 1.0, 1.0, 1.0, 1.0, 1.0, 1.0, 1.0, 1.0, 1.0, 1.0, 1.0, 1.0, 1.0, 1.0, 1.0, 1.0, 1.0, 1.0, 1.0, 1.0, 1.0, 1.0, 1.0, 1.0, 1.0, 1.0, 1.0, 1.0, 1.0, 1.0, 1.0, 1.0, 1.0, 1.0, 1.0, 1.0, 1.0, 1.0, 1.0, 1.0, 1.0, 1.0, 1.0, 1.0, 1.0, 1.0, 1.0, 1.0, 1.0, 1.0, 1.0, 1.0, 1.0, 1.0, 1.0, 1.0, 1.0, 1.0, 1.0, 1.0, 1.0, 1.0, 1.0, 1.0, 1.0, 1.0, 1.0, 1.0, 1.0, 1.0, 1.0, 1.0, 1.0, 1.0, 1.0, 1.0, 1.0, 1.0, 1.0, 1.0, 1.0, 1.0, 1.0, 1.0, 1.0, 1.0, 1.0, 1.0, 1.0, 1.0, 1.0, 1.0, 1.0, 1.0, 1.0, 1.0, 1.0, 1.0, 1.0, 1.0, 1.0, 1.0, 1.0, 1.0, 1.0, 1.0, 1.0, 1.0, 1.0, 1.0, 1.0, 1.0, 1.0, 1.0, 1.0, 1.0, 1.0, 1.0, 1.0, 1.0, 1.0, 1.0, 1.0, 1.0, 1.0, 1.0, 1.0, 1.0, 1.0, 1.0, 1.0, 1.0, 1.0, 1.0, 1.0, 1.0], "Y"=array[280 elements]}]
  in  "dead time":dbl=3.7e-08
  out "Optical Depth":cluster{"Y":dbl[], "Y":dbl[]}[](graph) caption="XY Graph"
  out "RingBuffer offline far":dbl[][](array[numeric])
  out "RingBuffer aerosol far":dbl[][](array[numeric])
  in  "Weather":T3(tab)=enum."Pulse Energy (Micro Joule)"
  out "Temperature (C)":dbl(graph)=28.964285714285708
  out "Pressure (mb)":dbl(graph)=984.5192307692307
  out "Relative Humdity (%)":dbl(graph)=41.800976800976805
  out "Pulse Energy (Micro Joule)":cluster{dbl}(graph)={3.49579831932773}
  in  "PRF (kHz)":dbl=7.0
  in  "energy scale":dbl=0.0425
  out "?":cluster{"mean":dbl, "mean":dbl}(graph)={"mean"=175840.0, "mean"=0.0}
  out "Index":i32=155894
  out "Aerosol Smoothed":dbl[](array[numeric])=[58.75133333333335, 82.08466666666669, 102.96800000000003, 124.66800000000003, 147.00133333333338, 168.7846666666667, 198.8846666666667, 228.95133333333334, 271.7346666666666, 312.93466666666666, 334.76800000000003, 367.4346666666667, 413.40133333333335, 451.568, 479.36800000000005, 518.1346666666667, 559.0846666666667, 583.3513333333335, 611.5680000000002, 624.4680000000001, 610.8013333333336, 611.4013333333335, 596.2180000000002, 508.9846666666668, 396.1846666666667, 318.7513333333333, 281.80133333333333, 248.368, 217.13466666666665, 209.48466666666667, 216.31799999999998, 226.46800000000002, 228.58466666666666, 226.28466666666668, 211.25133333333338, 190.31800000000004, 180.68466666666671, 165.2346666666667, 146.15133333333335, 138.6346666666667, 137.95133333333337, 126.90133333333337, 119.8846666666667, 116.50133333333336, 108.25133333333336, 103.21800000000003, 102.91800000000003, 109.06800000000004, 102.80133333333336, 91.21800000000002, 89.66800000000003, 89.3846666666667, 88.4846666666667, 81.01800000000003, 73.95133333333337, 69.06800000000003, 71.2346666666667, 73.55133333333336, 74.41800000000003, 6288.268000000001, 23020.484666666664, 37694.78466666666, 33736.21799999999, 15942.484666666667, 3214.8013333333342, 85.78466666666668, -4.915333333333331, -8.948666666666664, -6.448666666666664, -9.21533333333333, -7.581999999999997, -5.931999999999998, -4.998666666666664, -1.0153333333333308, -5.715333333333331, -11.931999999999999, -3.981999999999998, 2.7346666666666692, -2.8153333333333306, -8.46533333333333, -8.748666666666663, -3.7153333333333305, -5.831999999999997, -8.71533333333333, -4.881999999999997, -4.181999999999998, -8.431999999999999, -4.165333333333331, 4.534666666666669, 2.9346666666666694, 3.701333333333336, 9.418000000000003, 6.734666666666669, 11.168000000000003, 17.168000000000003, 16.418000000000003, 14.73466666666667, 8.418000000000003, 8.368000000000002, 11.751333333333335, 2.8180000000000027, 0.05133333333333567, 1.1513333333333358, -2.0153333333333308, 1.5846666666666693, -1.148666666666664, -4.381999999999998, 3.0346666666666695, 5.701333333333336, -0.8319999999999974, -0.9486666666666641, 1.3180000000000027, -2.1319999999999975, -4.431999999999997, -0.3153333333333306, 1.9180000000000026, -1.2653333333333308, -4.315333333333331, 0.001333333333335851, 5.668000000000003, 5.434666666666669, -0.7653333333333308, -2.9819999999999975, -0.03199999999999742, 0.6013333333333359, 2.3180000000000027, 3.618000000000003, 5.451333333333336, 4.234666666666669, -2.6819999999999973, -11.36533333333333, -7.298666666666664, 2.351333333333336, -0.24866666666666437, -6.865333333333331, -4.365333333333331, -2.1986666666666643, -7.281999999999997, -6.565333333333331, -3.831999999999997, -1.9819999999999975, 4.634666666666669, 3.3846666666666687, 1.4346666666666692, -6.098666666666663, -8.41533333333333, -1.3319999999999974, -5.415333333333331, -5.998666666666664, -1.8486666666666642, -1.0153333333333308, -0.6486666666666642, 1.9846666666666692, 2.5680000000000023, 6.468000000000003, 3.5846666666666698, -1.448666666666664, -7.248666666666663, -5.11533333333333, 5.618000000000002, 8.28466666666667, 4.03466666666667, -1.8653333333333306, -6.1486666666666645, 3.668000000000002, 5.418000000000003, -7.131999999999998, -3.998666666666664, -5.148666666666664, -2.9153333333333302, 0.18466666666666942, -8.281999999999996, -2.8819999999999975, 5.0180000000000025, -0.04866666666666419, -4.998666666666664, -3.6986666666666643, -4.931999999999997, -4.815333333333331, 0.9180000000000026, 0.051333333333335895, -7.098666666666665, -9.61533333333333, -6.048666666666664, -11.61533333333333, -5.831999999999997, -1.8319999999999976, -4.615333333333331, -3.3153333333333306, -4.2319999999999975, -0.8986666666666641, -0.48199999999999743, 2.9346666666666694, 3.101333333333336, 1.0346666666666693, 0.7846666666666693, -0.9319999999999975, -1.1653333333333307, -3.6819999999999977, -5.61533333333333, -5.448666666666664, -4.648666666666664, -3.5153333333333308, -2.548666666666664, -2.1153333333333304, -3.3153333333333306, -4.015333333333331, -1.548666666666664, -4.698666666666664, -6.681999999999997, -6.048666666666664, -5.298666666666664, -2.6653333333333307, -4.698666666666664, -5.498666666666664, -5.798666666666664, -8.181999999999997, -6.36533333333333, 0.051333333333335895, -0.9319999999999975, -2.715333333333331, 0.38466666666666927, 0.9013333333333359, 1.1180000000000025, -0.9819999999999973, -0.6319999999999972, 6.234666666666669, 3.9346666666666694, -5.881999999999998, -8.131999999999998, -7.831999999999997, -5.931999999999997, -2.0986666666666642, -0.848666666666664, -3.765333333333331, -6.081999999999997, -1.3653333333333306, 1.101333333333336, 0.7846666666666693, -1.348666666666664, 0.1680000000000026, 4.001333333333336, -0.39866666666666406, -0.48199999999999754, -2.531999999999998, -8.331999999999997, -5.098666666666664, -6.698666666666664, -2.2819999999999974, 2.418000000000003, -0.2653333333333308, -3.831999999999997, -0.9153333333333307, 4.318000000000002, -2.8319999999999976, -6.098666666666665, 2.268000000000003, 3.2346666666666697, -1.8653333333333306, 0.1680000000000026, 2.418000000000003, 5.401333333333336, 12.084666666666669, 9.151333333333335, 4.051333333333336, 0.951333333333336, -2.098666666666664, -2.3653333333333304, -6.398666666666664, -4.131999999999998, -1.7653333333333308, -2.348666666666664, -6.165333333333331, -5.381999999999998, -4.331999999999997, -2.5319999999999974, 2.3180000000000023]
  out "Off-Line  Bin Readings":dbl[](array[numeric])=[907.0, 983.0, 936.0, 968.0, 1058.0, 1048.0, 1078.0, 1121.0, 1171.0, 1196.0, 1260.0, 1232.0, 1317.0, 1311.0, 1458.0, 1316.0, 1429.0, 1416.0, 1484.0, 1551.0, 1493.0, 1523.0, 1472.0, 1457.0, 1350.0, 1231.0, 1196.0, 1203.0, 1131.0, 1064.0, 1117.0, 1113.0, 1111.0, 1124.0, 1151.0, 1048.0, 1058.0, 1038.0, 949.0, 1026.0, 970.0, 1033.0, 956.0, 1042.0, 983.0, 981.0, 998.0, 976.0, 980.0, 943.0, 997.0, 964.0, 975.0, 961.0, 987.0, 917.0, 942.0, 980.0, 946.0, 949.0, 15670.0, 43906.0, 41123.0, 12026.0, 1493.0, 900.0, 857.0, 812.0, 913.0, 819.0, 875.0, 881.0, 895.0, 852.0, 870.0, 861.0, 875.0, 899.0, 898.0, 877.0, 871.0, 917.0, 833.0, 927.0, 890.0, 897.0, 861.0, 840.0, 878.0, 880.0, 896.0, 885.0, 900.0, 834.0, 899.0, 893.0, 856.0, 860.0, 939.0, 885.0, 863.0, 906.0, 936.0, 880.0, 878.0, 845.0, 908.0, 824.0, 872.0, 878.0, 872.0, 887.0, 869.0, 888.0, 896.0, 903.0, 850.0, 882.0, 875.0, 889.0, 935.0, 900.0, 856.0, 884.0, 807.0, 854.0, 869.0, 935.0, 894.0, 874.0, 883.0, 894.0, 854.0, 943.0, 884.0, 834.0, 871.0, 824.0, 848.0, 893.0, 897.0, 902.0, 854.0, 923.0, 900.0, 880.0, 906.0, 866.0, 872.0, 844.0, 895.0, 883.0, 889.0, 921.0, 877.0, 896.0, 894.0, 833.0, 899.0, 881.0, 902.0, 887.0, 847.0, 900.0, 865.0, 864.0, 876.0, 871.0, 891.0, 859.0, 902.0, 922.0, 882.0, 844.0, 927.0, 908.0, 855.0, 890.0, 900.0, 872.0, 889.0, 868.0, 869.0, 829.0, 847.0, 877.0, 880.0, 813.0, 881.0, 884.0, 862.0, 839.0, 892.0, 924.0, 913.0, 874.0, 859.0, 888.0, 854.0, 846.0, 819.0, 877.0, 806.0, 879.0, 923.0, 864.0, 894.0, 885.0, 851.0, 850.0, 860.0, 855.0, 867.0, 903.0, 876.0, 886.0, 895.0, 847.0, 885.0, 886.0, 811.0, 878.0, 843.0, 890.0, 839.0, 871.0, 904.0, 930.0, 922.0, 882.0, 885.0, 859.0, 851.0, 916.0, 886.0, 850.0, 904.0, 900.0, 873.0, 877.0, 911.0, 897.0, 874.0, 972.0, 879.0, 877.0, 795.0, 882.0, 864.0, 857.0, 849.0, 887.0, 880.0, 903.0, 915.0, 880.0, 842.0, 882.0, 900.0, 841.0, 899.0, 840.0, 832.0, 907.0, 807.0, 913.0, 915.0, 876.0, 849.0, 862.0, 911.0, 860.0, 850.0, 921.0, 895.0, 877.0, 890.0, 885.0, 931.0]
  out "Off-Line Smoothed":dbl[](array[numeric])=[57.090888888888884, 74.17144444444443, 92.36033333333333, 114.02422222222219, 136.31588888888885, 159.0825555555555, 187.16033333333328, 214.13533333333334, 243.48255555555556, 273.4047777777778, 301.6242222222222, 336.4464444444444, 369.40199999999993, 393.0825555555555, 419.5436666666666, 452.3714444444444, 488.51588888888887, 521.988111111111, 549.4381111111111, 564.2908888888887, 565.463111111111, 565.9908888888888, 538.7714444444443, 451.2242222222221, 348.0575555555555, 283.18255555555555, 248.152, 223.98255555555556, 211.1658888888889, 211.36033333333336, 217.64088888888892, 224.36866666666668, 227.09922222222224, 223.40200000000004, 211.63811111111116, 190.5658888888889, 173.00755555555554, 161.65755555555552, 149.29922222222217, 136.59088888888886, 132.37977777777775, 128.4242222222222, 119.41033333333333, 114.30755555555554, 111.22144444444442, 108.34922222222221, 103.69922222222223, 100.75755555555557, 95.93811111111111, 89.59366666666668, 91.06588888888889, 88.42422222222223, 83.79088888888889, 79.87144444444445, 74.86866666666667, 70.78255555555556, 69.34366666666668, 73.06866666666666, 73.15477777777777, 1839.7353333333335, 9732.83811111111, 23207.90755555556, 31775.77144444445, 25937.44366666667, 11318.11033333334, 1920.7297777777792, 47.61588888888888, 4.190888888888889, 1.0519999999999987, 3.026999999999999, 2.13811111111111, 1.8158888888888878, 3.5686666666666653, 2.8547777777777767, 2.010333333333332, 1.0797777777777764, 2.1325555555555544, 1.3408888888888877, -0.19800000000000118, -0.08688888888889013, -0.5952222222222234, 1.0464444444444432, 2.574222222222221, 2.51311111111111, 1.9214444444444432, -1.2924444444444458, -4.289666666666668, -1.273000000000001, 1.674222222222221, 1.8158888888888876, 3.160333333333332, 13.640888888888892, 44.576999999999984, 127.74088888888888, 228.53811111111108, 272.5103333333333, 279.013111111111, 284.32144444444435, 276.063111111111, 243.49644444444436, 195.19366666666662, 143.827, 104.64366666666666, 80.34644444444442, 69.92699999999998, 66.52977777777775, 57.31588888888888, 46.56311111111111, 32.857555555555564, 20.124222222222222, 16.479777777777777, 14.171444444444445, 9.074222222222225, 4.004777777777778, 2.7575555555555544, 2.074222222222221, 1.6547777777777766, 3.6436666666666655, 5.26311111111111, 3.9603333333333324, 2.3103333333333325, 1.2103333333333322, 1.0964444444444432, 3.1131111111111096, 3.085333333333332, 0.7769999999999988, -0.31466666666666787, 2.1408888888888873, 2.2658888888888873, -0.9674444444444457, -1.089666666666668, -0.6702222222222234, -0.7007777777777789, -2.4952222222222233, -2.7285555555555567, 0.4519999999999988, 0.5381111111111099, 1.199222222222221, 0.46033333333333215, -3.134111111111112, -3.4063333333333343, 0.3658888888888878, 1.876999999999999, 1.2186666666666655, -0.9563333333333344, -0.8924444444444455, 1.0658888888888878, -1.3646666666666678, -2.5535555555555565, -0.53688888888889, -0.5952222222222233, -1.7646666666666677, 0.8714444444444434, 0.9686666666666655, -0.025777777777778954, -0.025777777777778954, 0.16033333333333216, -1.6702222222222236, -2.1341111111111126, -0.2868888888888901, 0.021444444444443267, -1.178555555555557, -1.7674444444444457, -1.889666666666668, -0.5230000000000012, 0.4936666666666655, -1.0424444444444456, -0.6480000000000012, -2.5452222222222236, -2.7063333333333346, 0.19922222222222108, -0.8313333333333345, -1.2563333333333344, 0.2047777777777766, -1.814666666666668, -3.803555555555557, -1.9980000000000013, -0.40077777777777895, -0.250777777777779, -1.7313333333333345, -0.9785555555555568, -1.0868888888888901, -4.342444444444445, -3.089666666666668, -3.1341111111111126, -2.0591111111111124, -1.2202222222222234, -0.30911111111111245, 2.346444444444443, -1.2618888888888902, -2.2091111111111124, 2.413111111111111, 1.4325555555555556, -0.5313333333333345, 0.4186666666666655, -0.5730000000000012, -2.2924444444444454, -0.44800000000000106, -0.03966666666666785, -1.6980000000000013, 0.3158888888888877, -1.517444444444446, -2.803555555555557, 1.7603333333333322, 1.7908888888888876, -0.08966666666666784, -0.725777777777779, -0.9924444444444457, -0.2868888888888901, 0.3047777777777766, -0.7285555555555567, -0.6591111111111123, 1.5547777777777765, -0.5146666666666678, -3.256333333333335, -2.4785555555555567, -0.15633333333333455, 0.09644444444444322, 0.08533333333333215, -0.9174444444444455, -0.44244444444444553, 0.051999999999998825, -2.3535555555555567, -1.4257777777777791, 0.03255555555555435, -0.061888888888890076, -0.24244444444444563, -0.0007777777777789319, -2.5535555555555574, -3.3841111111111126, -0.46466666666666784, -0.023000000000001186, -0.45077777777777894, 0.7519999999999989, 1.285333333333332, 0.46033333333333215, -0.5841111111111122, -0.8535555555555567, 0.4575555555555544, 0.8353333333333322, 2.049222222222221, 2.024222222222221, 0.6769999999999987, 1.435333333333332, -0.20911111111111236, -2.9202222222222236, -2.0535555555555565, 0.299222222222221, 1.6769999999999987, 0.2964444444444432, -0.21188888888889013, -1.6841111111111124, -2.18688888888889, 1.6686666666666654, -2.0229999999999997, -6.050777777777777, -3.9674444444444457, -2.3202222222222235, -0.9368888888888901, 0.043666666666665466, 1.3797777777777767, 0.5964444444444432, 0.6992222222222209, 0.9269999999999987, 1.3047777777777767, 2.1047777777777767, 1.876999999999999, 1.8797777777777767, 0.4492222222222211, 0.10477777777777658, 1.6769999999999987, 0.48533333333333206, -0.46744444444444566, 0.32699999999999885, -0.7341111111111123, 1.1686666666666654, 0.4797777777777765]
  out "On-Line  Smoothed":dbl[](array[numeric])=[44.907111111111114, 56.193222222222225, 67.41822222222223, 78.61822222222223, 88.15155555555556, 97.32933333333338, 106.34600000000009, 114.26266666666675, 122.14322222222228, 132.25988888888895, 140.65988888888893, 143.0043333333334, 145.21266666666673, 148.5821111111112, 154.2043333333334, 161.39322222222228, 162.48488888888892, 164.15433333333337, 166.7793333333334, 160.32655555555561, 155.2793333333334, 148.5626666666667, 134.06266666666673, 109.11266666666671, 80.62655555555557, 65.04599999999999, 55.596000000000004, 47.179333333333346, 41.726555555555564, 40.60433333333334, 42.80155555555556, 41.89044444444445, 40.28488888888889, 42.79600000000001, 41.229333333333344, 33.54600000000001, 28.646000000000008, 24.754333333333342, 23.03211111111112, 22.498777777777786, 22.15155555555556, 19.518222222222228, 17.657111111111117, 19.18211111111112, 17.382111111111115, 15.368222222222226, 12.068222222222225, 11.334888888888893, 11.721000000000004, 9.67377777777778, 8.97377777777778, 12.354333333333336, 11.915444444444448, 9.754333333333337, 10.304333333333336, 10.098777777777782, 8.62377777777778, 6.598777777777778, 7.518222222222224, 247.59044444444444, 1300.846, 3214.10988888889, 4426.404333333336, 3520.465444444446, 1464.10988888889, 217.17100000000025, 4.809888888888891, 1.173777777777779, -1.19011111111111, -1.6039999999999988, 0.04322222222222333, -0.7845555555555545, -1.451222222222221, -0.7234444444444433, 0.8210000000000011, 0.9543333333333344, 1.532111111111112, 0.571000000000001, -2.2623333333333324, -1.5428888888888879, -0.18455555555555445, 2.8793333333333337, 2.146000000000001, -0.9539999999999988, -0.49288888888888777, -1.46511111111111, -3.19011111111111, -2.3095555555555545, 0.3043333333333345, 2.0904444444444454, 1.95988888888889, 0.5793333333333344, 2.832111111111112, 9.712666666666669, 20.459888888888905, 26.393222222222246, 26.88766666666669, 28.80155555555558, 26.765444444444462, 20.99877777777779, 16.718222222222227, 12.776555555555559, 11.08766666666667, 7.726555555555558, 3.4765555555555565, 5.109888888888891, 4.476555555555558, 2.071000000000001, 1.0376666666666678, 1.6043333333333345, 2.7460000000000013, 2.357111111111112, 1.30988888888889, 1.9543333333333344, 1.4210000000000012, -1.5706666666666655, -2.59011111111111, -1.66511111111111, -1.3873333333333322, -0.09566666666666557, 0.8210000000000011, 0.06266666666666779, -1.8317777777777766, -2.8928888888888875, -0.3873333333333322, 0.5071111111111123, -0.56511111111111, -1.1567777777777768, -0.69011111111111, -0.1012222222222211, -1.612333333333332, -1.84011111111111, -0.04288888888888778, -0.44844444444444337, -3.351222222222222, -4.0873333333333335, -0.6373333333333322, 0.4404444444444455, -0.23455555555555446, -1.0067777777777767, -1.9678888888888877, -0.94011111111111, -0.06233333333333223, -1.1651111111111099, -2.759555555555554, -2.0234444444444435, -2.3817777777777764, -0.9901111111111098, 1.4126666666666678, -1.6873333333333322, -4.287333333333333, -3.517888888888888, -0.02344444444444349, 0.14600000000000102, 1.1598888888888899, 1.5182222222222232, -2.620666666666666, -1.5706666666666655, 0.04322222222222333, 0.3293333333333344, 0.6821111111111122, 0.20988888888889, 1.3737777777777789, 0.16822222222222316, -1.3345555555555544, -0.39011111111110996, 0.46544444444444555, -0.31511111111111, -1.8678888888888876, -0.8651111111111099, 0.5543333333333345, -0.9512222222222211, -0.045666666666665634, 1.3043333333333345, -0.017888888888887775, -0.8484444444444433, -1.3706666666666656, -0.37344444444444336, -0.6234444444444434, -1.9484444444444433, -2.2706666666666653, -1.503999999999999, -0.015111111111110076, -0.5956666666666656, -2.5345555555555546, -0.7678888888888877, -1.153999999999999, 0.12655555555555664, 1.698777777777779, -1.0401111111111099, -1.39011111111111, -0.5123333333333322, 0.36822222222222334, 0.40988888888888997, 0.30988888888889, 1.0210000000000012, -0.059555555555554474, 0.05988888888888999, 2.0682222222222233, 2.4376666666666678, 2.4432222222222233, 1.0654444444444455, 0.015444444444445558, 0.8071111111111122, -0.24566666666666548, -2.0123333333333324, -2.326222222222221, -2.0206666666666653, -0.7178888888888878, -1.8595555555555543, -1.6178888888888876, -1.2595555555555547, -2.1095555555555547, -1.3428888888888877, 0.16822222222222327, 1.3321111111111121, 2.126555555555557, 2.4404444444444455, 0.14322222222222336, 0.06544444444444553, -0.7595555555555544, -2.276222222222221, -1.3817777777777767, -0.3178888888888878, -1.4178888888888876, -0.3067777777777765, -0.07899999999999885, -2.870666666666666, -2.0234444444444435, 0.023777777777778897, 1.3793333333333346, -0.9901111111111099, -1.8678888888888878, -0.6539999999999988, -0.26788888888888773, 0.6071111111111123, -0.9428888888888878, -2.9595555555555544, -1.4345555555555545, 0.5265555555555567, -0.8873333333333321, 0.07655555555555682, -0.35399999999999876, -0.22899999999999876, -0.1289999999999989, -1.228999999999999, -0.28733333333333216, -1.0706666666666655, -1.3734444444444434, -0.8678888888888878, 0.15433333333333443, -0.028999999999998888, -1.5123333333333322, -0.4206666666666655, 1.9571111111111121, 1.071000000000001, -0.06511111111111, 0.4515555555555567, 0.55988888888889, 2.4321111111111122, 2.2571111111111124, -0.9956666666666655, -1.2984444444444434, 0.7015555555555566, 2.05988888888889, 0.5154444444444456, -1.4428888888888878, -0.6178888888888878, -0.8956666666666655, -1.3623333333333323, 0.7571111111111123, 0.8821111111111123, -1.2123333333333324, -2.759555555555554, -1.276222222222221, 0.6960000000000011, -1.1234444444444434]
  out "On-Line Bin Readings":dbl[](array[numeric])=[953.0, 932.0, 968.0, 971.0, 975.0, 997.0, 991.0, 1059.0, 971.0, 988.0, 1028.0, 1020.0, 1069.0, 1035.0, 1043.0, 1018.0, 1035.0, 1069.0, 1083.0, 1089.0, 1060.0, 1023.0, 1021.0, 1048.0, 972.0, 992.0, 974.0, 906.0, 903.0, 919.0, 917.0, 925.0, 915.0, 918.0, 887.0, 920.0, 946.0, 913.0, 893.0, 887.0, 914.0, 891.0, 882.0, 949.0, 876.0, 902.0, 942.0, 878.0, 914.0, 864.0, 926.0, 886.0, 922.0, 860.0, 914.0, 859.0, 897.0, 875.0, 929.0, 877.0, 2906.0, 7078.0, 6779.0, 2294.0, 918.0, 848.0, 887.0, 972.0, 866.0, 895.0, 872.0, 847.0, 921.0, 891.0, 855.0, 846.0, 904.0, 879.0, 902.0, 864.0, 914.0, 906.0, 908.0, 884.0, 881.0, 870.0, 884.0, 855.0, 861.0, 867.0, 952.0, 810.0, 927.0, 880.0, 858.0, 884.0, 949.0, 892.0, 888.0, 870.0, 919.0, 878.0, 900.0, 935.0, 921.0, 872.0, 852.0, 842.0, 873.0, 860.0, 923.0, 880.0, 837.0, 863.0, 911.0, 882.0, 814.0, 830.0, 929.0, 939.0, 859.0, 937.0, 870.0, 874.0, 843.0, 933.0, 866.0, 852.0, 920.0, 921.0, 894.0, 837.0, 870.0, 929.0, 817.0, 861.0, 882.0, 856.0, 862.0, 919.0, 903.0, 913.0, 866.0, 861.0, 907.0, 842.0, 858.0, 932.0, 876.0, 903.0, 852.0, 852.0, 899.0, 914.0, 904.0, 813.0, 845.0, 928.0, 865.0, 871.0, 852.0, 876.0, 884.0, 881.0, 936.0, 913.0, 862.0, 887.0, 857.0, 903.0, 889.0, 907.0, 831.0, 900.0, 949.0, 900.0, 893.0, 873.0, 853.0, 865.0, 885.0, 873.0, 871.0, 892.0, 930.0, 883.0, 899.0, 880.0, 896.0, 879.0, 850.0, 853.0, 876.0, 850.0, 923.0, 889.0, 855.0, 865.0, 873.0, 913.0, 846.0, 891.0, 875.0, 911.0, 893.0, 884.0, 910.0, 914.0, 890.0, 891.0, 828.0, 851.0, 877.0, 895.0, 877.0, 881.0, 845.0, 875.0, 839.0, 928.0, 835.0, 865.0, 892.0, 913.0, 880.0, 870.0, 880.0, 881.0, 874.0, 903.0, 827.0, 856.0, 893.0, 889.0, 835.0, 864.0, 897.0, 917.0, 907.0, 851.0, 883.0, 855.0, 895.0, 870.0, 907.0, 906.0, 895.0, 899.0, 855.0, 877.0, 882.0, 873.0, 908.0, 877.0, 943.0, 864.0, 891.0, 870.0, 865.0, 950.0, 865.0, 893.0, 906.0, 881.0, 911.0, 858.0, 898.0, 825.0, 861.0, 880.0, 902.0, 893.0, 902.0, 921.0, 889.0, 878.0, 886.0, 872.0, 911.0]
  out "Range Corrected Altitude Array":dbl[](array[numeric])=[5625.0, 22500.0, 50625.0, 90000.0, 140625.0, 202500.0, 275625.0, 360000.0, 455625.0, 562500.0, 680625.0, 810000.0, 950625.0, 1102500.0, 1265625.0, 1440000.0, 1625625.0, 1822500.0, 2030625.0, 2250000.0, 2480625.0, 2722500.0, 2975625.0, 3240000.0, 3515625.0, 3802500.0, 4100625.0, 4410000.0, 4730625.0, 5062500.0, 5405625.0, 5760000.0, 6125625.0, 6502500.0, 6890625.0, 7290000.0, 7700625.0, 8122500.0, 8555625.0, 9000000.0, 9455625.0, 9922500.0, 10400625.0, 10890000.0, 11390625.0, 11902500.0, 12425625.0, 12960000.0, 13505625.0, 14062500.0, 14630625.0, 15210000.0, 15800625.0, 16402500.0, 17015625.0, 17640000.0, 18275625.0, 18922500.0, 19580625.0, 20250000.0, 20930625.0, 21622500.0, 22325625.0, 23040000.0, 23765625.0, 24502500.0, 25250625.0, 26010000.0, 26780625.0, 27562500.0, 28355625.0, 29160000.0, 29975625.0, 30802500.0, 31640625.0, 32490000.0, 33350625.0, 34222500.0, 35105625.0, 36000000.0, 36905625.0, 37822500.0, 38750625.0, 39690000.0, 40640625.0, 41602500.0, 42575625.0, 43560000.0, 44555625.0, 45562500.0, 46580625.0, 47610000.0, 48650625.0, 49702500.0, 50765625.0, 51840000.0, 52925625.0, 54022500.0, 55130625.0, 56250000.0, 57380625.0, 58522500.0, 59675625.0, 60840000.0, 62015625.0, 63202500.0, 64400625.0, 65610000.0, 66830625.0, 68062500.0, 69305625.0, 70560000.0, 71825625.0, 73102500.0, 74390625.0, 75690000.0, 77000625.0, 78322500.0, 79655625.0, 81000000.0, 82355625.0, 83722500.0, 85100625.0, 86490000.0, 87890625.0, 89302500.0, 90725625.0, 92160000.0, 93605625.0, 95062500.0, 96530625.0, 98010000.0, 99500625.0, 101002500.0, 102515625.0, 104040000.0, 105575625.0, 107122500.0, 108680625.0, 110250000.0, 111830625.0, 113422500.0, 115025625.0, 116640000.0, 118265625.0, 119902500.0, 121550625.0, 123210000.0, 124880625.0, 126562500.0, 128255625.0, 129960000.0, 131675625.0, 133402500.0, 135140625.0, 136890000.0, 138650625.0, 140422500.0, 142205625.0, 144000000.0, 145805625.0, 147622500.0, 149450625.0, 151290000.0, 153140625.0, 155002500.0, 156875625.0, 158760000.0, 160655625.0, 162562500.0, 164480625.0, 166410000.0, 168350625.0, 170302500.0, 172265625.0, 174240000.0, 176225625.0, 178222500.0, 180230625.0, 182250000.0, 184280625.0, 186322500.0, 188375625.0, 190440000.0, 192515625.0, 194602500.0, 196700625.0, 198810000.0, 200930625.0, 203062500.0, 205205625.0, 207360000.0, 209525625.0, 211702500.0, 213890625.0, 216090000.0, 218300625.0, 220522500.0, 222755625.0, 225000000.0, 227255625.0, 229522500.0, 231800625.0, 234090000.0, 236390625.0, 238702500.0, 241025625.0, 243360000.0, 245705625.0, 248062500.0, 250430625.0, 252810000.0, 255200625.0, 257602500.0, 260015625.0, 262440000.0, 264875625.0, 267322500.0, 269780625.0, 272250000.0, 274730625.0, 277222500.0, 279725625.0, 282240000.0, 284765625.0, 287302500.0, 289850625.0, 292410000.0, 294980625.0, 297562500.0, 300155625.0, 302760000.0, 305375625.0, 308002500.0, 310640625.0, 313290000.0, 315950625.0, 318622500.0, 321305625.0, 324000000.0, 326705625.0, 329422500.0, 332150625.0, 334890000.0, 337640625.0, 340402500.0, 343175625.0, 345960000.0, 348755625.0, 351562500.0, 354380625.0, 357210000.0, 360050625.0, 362902500.0, 365765625.0, 368640000.0, 371525625.0, 374422500.0, 377330625.0, 380250000.0, 383180625.0, 386122500.0, 389075625.0, 392040000.0, 395015625.0, 398002500.0, 401000625.0, 404010000.0, 407030625.0, 410062500.0, 413105625.0, 416160000.0, 419225625.0, 422302500.0, 425390625.0, 428490000.0, 431600625.0, 434722500.0, 437855625.0, 441000000.0]
  out "Altitude Array (km)":dbl[](array[numeric])=[0.075, 0.15, 0.22499999999999998, 0.3, 0.375, 0.45, 0.5249999999999999, 0.6, 0.6749999999999999, 0.7499999999999999, 0.825, 0.8999999999999999, 0.9749999999999999, 1.05, 1.125, 1.2, 1.275, 1.3499999999999999, 1.4249999999999998, 1.5, 1.575, 1.65, 1.7249999999999999, 1.7999999999999998, 1.8749999999999998, 1.95, 2.025, 2.1, 2.1750000000000003, 2.25, 2.325, 2.4, 2.475, 2.5500000000000003, 2.625, 2.7, 2.775, 2.85, 2.9250000000000003, 3.0, 3.075, 3.15, 3.225, 3.3000000000000003, 3.375, 3.45, 3.525, 3.6, 3.675, 3.75, 3.825, 3.9, 3.975, 4.05, 4.125, 4.2, 4.275, 4.35, 4.425, 4.5, 4.575, 4.65, 4.725, 4.8, 4.875, 4.95, 5.025, 5.1, 5.175, 5.25, 5.325, 5.4, 5.475, 5.55, 5.625, 5.7, 5.775, 5.85, 5.925, 6.0, 6.075, 6.15, 6.225, 6.3, 6.375, 6.45, 6.525, 6.6, 6.675, 6.75, 6.825, 6.9, 6.975, 7.05, 7.125, 7.2, 7.2749999999999995, 7.35, 7.425, 7.5, 7.575, 7.6499999999999995, 7.725, 7.8, 7.875, 7.95, 8.024999999999999, 8.1, 8.174999999999999, 8.249999999999998, 8.325, 8.399999999999999, 8.475, 8.549999999999999, 8.624999999999998, 8.7, 8.774999999999999, 8.85, 8.924999999999999, 8.999999999999998, 9.075, 9.149999999999999, 9.225, 9.299999999999999, 9.374999999999998, 9.45, 9.524999999999999, 9.6, 9.674999999999999, 9.749999999999998, 9.825, 9.899999999999999, 9.975, 10.049999999999999, 10.124999999999998, 10.2, 10.274999999999999, 10.35, 10.424999999999999, 10.499999999999998, 10.575, 10.649999999999999, 10.725, 10.799999999999999, 10.874999999999998, 10.95, 11.024999999999999, 11.1, 11.174999999999999, 11.249999999999998, 11.325, 11.399999999999999, 11.475, 11.549999999999999, 11.624999999999998, 11.7, 11.774999999999999, 11.85, 11.924999999999999, 11.999999999999998, 12.075, 12.149999999999999, 12.225, 12.299999999999999, 12.374999999999998, 12.45, 12.524999999999999, 12.6, 12.674999999999999, 12.749999999999998, 12.825, 12.899999999999999, 12.975, 13.049999999999999, 13.124999999999998, 13.2, 13.274999999999999, 13.35, 13.424999999999999, 13.499999999999998, 13.575, 13.649999999999999, 13.725, 13.799999999999999, 13.874999999999998, 13.95, 14.024999999999999, 14.1, 14.174999999999999, 14.249999999999998, 14.325, 14.399999999999999, 14.474999999999998, 14.549999999999999, 14.624999999999998, 14.7, 14.774999999999999, 14.849999999999998, 14.924999999999999, 14.999999999999998, 15.075, 15.149999999999999, 15.224999999999998, 15.299999999999999, 15.374999999999998, 15.45, 15.524999999999999, 15.599999999999998, 15.674999999999999, 15.749999999999998, 15.825, 15.899999999999999, 15.974999999999998, 16.05, 16.125, 16.2, 16.275, 16.349999999999998, 16.424999999999997, 16.5, 16.575, 16.65, 16.724999999999998, 16.799999999999997, 16.875, 16.95, 17.025, 17.099999999999998, 17.174999999999997, 17.25, 17.325, 17.4, 17.474999999999998, 17.549999999999997, 17.625, 17.7, 17.775, 17.849999999999998, 17.924999999999997, 18.0, 18.075, 18.15, 18.224999999999998, 18.299999999999997, 18.375, 18.45, 18.525, 18.599999999999998, 18.674999999999997, 18.75, 18.825, 18.9, 18.974999999999998, 19.049999999999997, 19.125, 19.2, 19.275, 19.349999999999998, 19.424999999999997, 19.5, 19.575, 19.65, 19.724999999999998, 19.799999999999997, 19.875, 19.95, 20.025, 20.099999999999998, 20.174999999999997, 20.25, 20.325, 20.4, 20.474999999999998, 20.549999999999997, 20.625, 20.7, 20.775, 20.849999999999998, 20.924999999999997, 21.0]
  in  "Instrument Control":T4(tab)
  out "Readings":T5={"OnLineTEC"=19.4780521, "OnLineLD"=0.155533209, "OffLineTEC"=18.5419254, "OffLineLD"=0.15476954, "EtalonTEC"=28.1040802, "TSOA-TEC"=20.0122318, "Pro8000"=TRUE, "OnLine TEC"=TRUE, "OnLine LD"=TRUE, "OffLine TEC"=TRUE, "OffLine LD"=TRUE, "Etalon TEC"=TRUE, "TSOA TEC"=TRUE} {"OffLineLD" format="%.4g"; "OnLineLD" format="%.4g"; "TSOA-TEC" format="%.3g"; "EtalonTEC" format="%.3g"; "OffLineTEC" format="%.3g"; "OnLineTEC" format="%.3g"}
  in  "Settings":T6={"Module"=enum."On Line TEC", "OnLineTEC"=19.473160000001542, "OnLineLD"=0.155, "OffLineTEC"=18.540920000001147, "OffLineLD"=0.155, "EtalonTEC"=28.1, "TSOA-TEC"=20.0} {"OffLineLD" min=0.0 max=0.175 step=0.001 format="%.3p"; "OnLineLD" min=0.0 max=0.175 step=0.001 format="%.3p"; "TSOA-TEC" format="%.2g"; "EtalonTEC" format="%.2g"; "OffLineTEC" min=0.0 max=30.0 step=0.1 format="%.3g"; "OnLineTEC" min=0.0 max=30.0 step=0.1 format="%.3g"}
  in  "Pulse B Polarity":enum32{"Low", "High"}(ring)=enum."High"
  in  "Pulse A Delay(ns)":u32=1040 min=80 max=327600
  in  "Pulse B Delay(ns)":u32=170000 min=80 max=327600 step=1
  in  "Accumulation Delay(ns)":u32=10 min=10 max=1270 step=1
  in  "Sync Pulse Polarity":enum32{"Low", "High"}(ring)=enum."High"
  in  "Pulse A Polarity":enum32{"Low", "High"}(ring)=enum."High"
  in  "Number of Bins":u32=280 min=2 max=4095 step=1
  in  "Number of Accumulates":u32=10000 min=1 max=32767 step=1
  in  "Time Resolution Per Bin(ns)":u32=500 min=5 max=1063 step=1
  out "WM Switch":bool
  in  "Cancel online":bool
  in  "Cancel Offline":bool
  in  "Lambda On Set (nm)":dbl=828.198 format="%.5f"
  out "Lambda On Read (nm)":dbl=828.1980499228852 format="%.5f"
  out "Lambda Off Read (nm)":dbl=828.2976847133127 format="%.5f"
  in  "Lambda Off Set (nm)":dbl=828.29765 format="%#.5f"
  in  "Bristol In":i32=5
  out "Bristol Out":i32=1
  in  "Online_Tol":dbl=5e-05 format="%#_15g"
  in  "Offline_Tol":dbl=0.0001 format="%#_15g"
  out "Wavelength Lock Online":bool=TRUE
  out "Wavelength Lock Offline":bool=TRUE
  out "WL Difference":dbl=4.992288518224086e-05 format="%_7g"
  out "WL Difference off":dbl=3.471331274340628e-05 format="%_7g"
  in  "calculate absorption cross sections":bool
  in  "Smoothing Range":dbl=150.0
  in  "Total DIAL Integration Time (Minutes)":i32=3
  in  "Data Reads (number of loops)":i32=1
  in  "Total Aerosol Integration Time (Minutes)":dbl=0.5
  in  "Scalar Wait Time (disabled)":u32
  out "Smoothed Bins":dbl=2.0
  in  "Ophir PM On/Off":bool=TRUE
  out "OphirPM":T7={"Ophir-Ref"=refnum, "Ophir-Device"=1000, "Ophir-Channel"=0}
  out "Average Diode Power":dbl(knob)=0.00104 scale=0.0..0.002 scale format="%.1p"
  out "Ophir Samples":i32=29
  in  "Switch Comm Port":refnum<visa-resource-name>="COM3"
  out "FF_On_Ref":refnum<file>
  out "FF_On_Ptr":i64=1455168 format="%.2p"
  out "FF_Off_Ref":refnum<file>
  out "FF_Off_Ptr":i64=1455168 format="%.2p"
  out "NF_On_Ref":refnum<file>
  out "NF_On_Ptr":i64=1455168 format="%.2p"
  out "NF_Off_Ref":refnum<file>
  out "NF_Off_Ptr":i64=1455168 format="%.2p"
  out "DataOpen":bool=TRUE
  out "File Path_Far Field (out)":string="D:\\Micropulse_DIAL_data\\170516FF\\17"
  out "File Path_Near Field (out)":string="D:\\Micropulse_DIAL_data\\170516NF\\17"
  in  "Data File DIR (in)":string="D:\\Micropulse_DIAL_data\\"
  in  "WS_On/Off":bool=TRUE
  in  "WS visa":refnum<visa-resource-name>="Weather"
  out "TRHP":T8={"Temp C"=28.964285714285708, "RelH %"=41.800976800976805, "Press hPa"=984.5192307692307, "AbH g/m^3"=10.347985347985349}
  in  "ADAM6018 IP":string="192.168.0.165"
  out "T_bench":sgl=23.39971
  in  "Port":u16=502
  in  "IP Address":string="192.168.0.165"
  out "ID_out":refnum<k5>
  in  "bins":u32=280 min=2 max=4095 step=1
  out "y offset":u32=10
  in  "ns scale":u32=500
  # "ADAM6018"
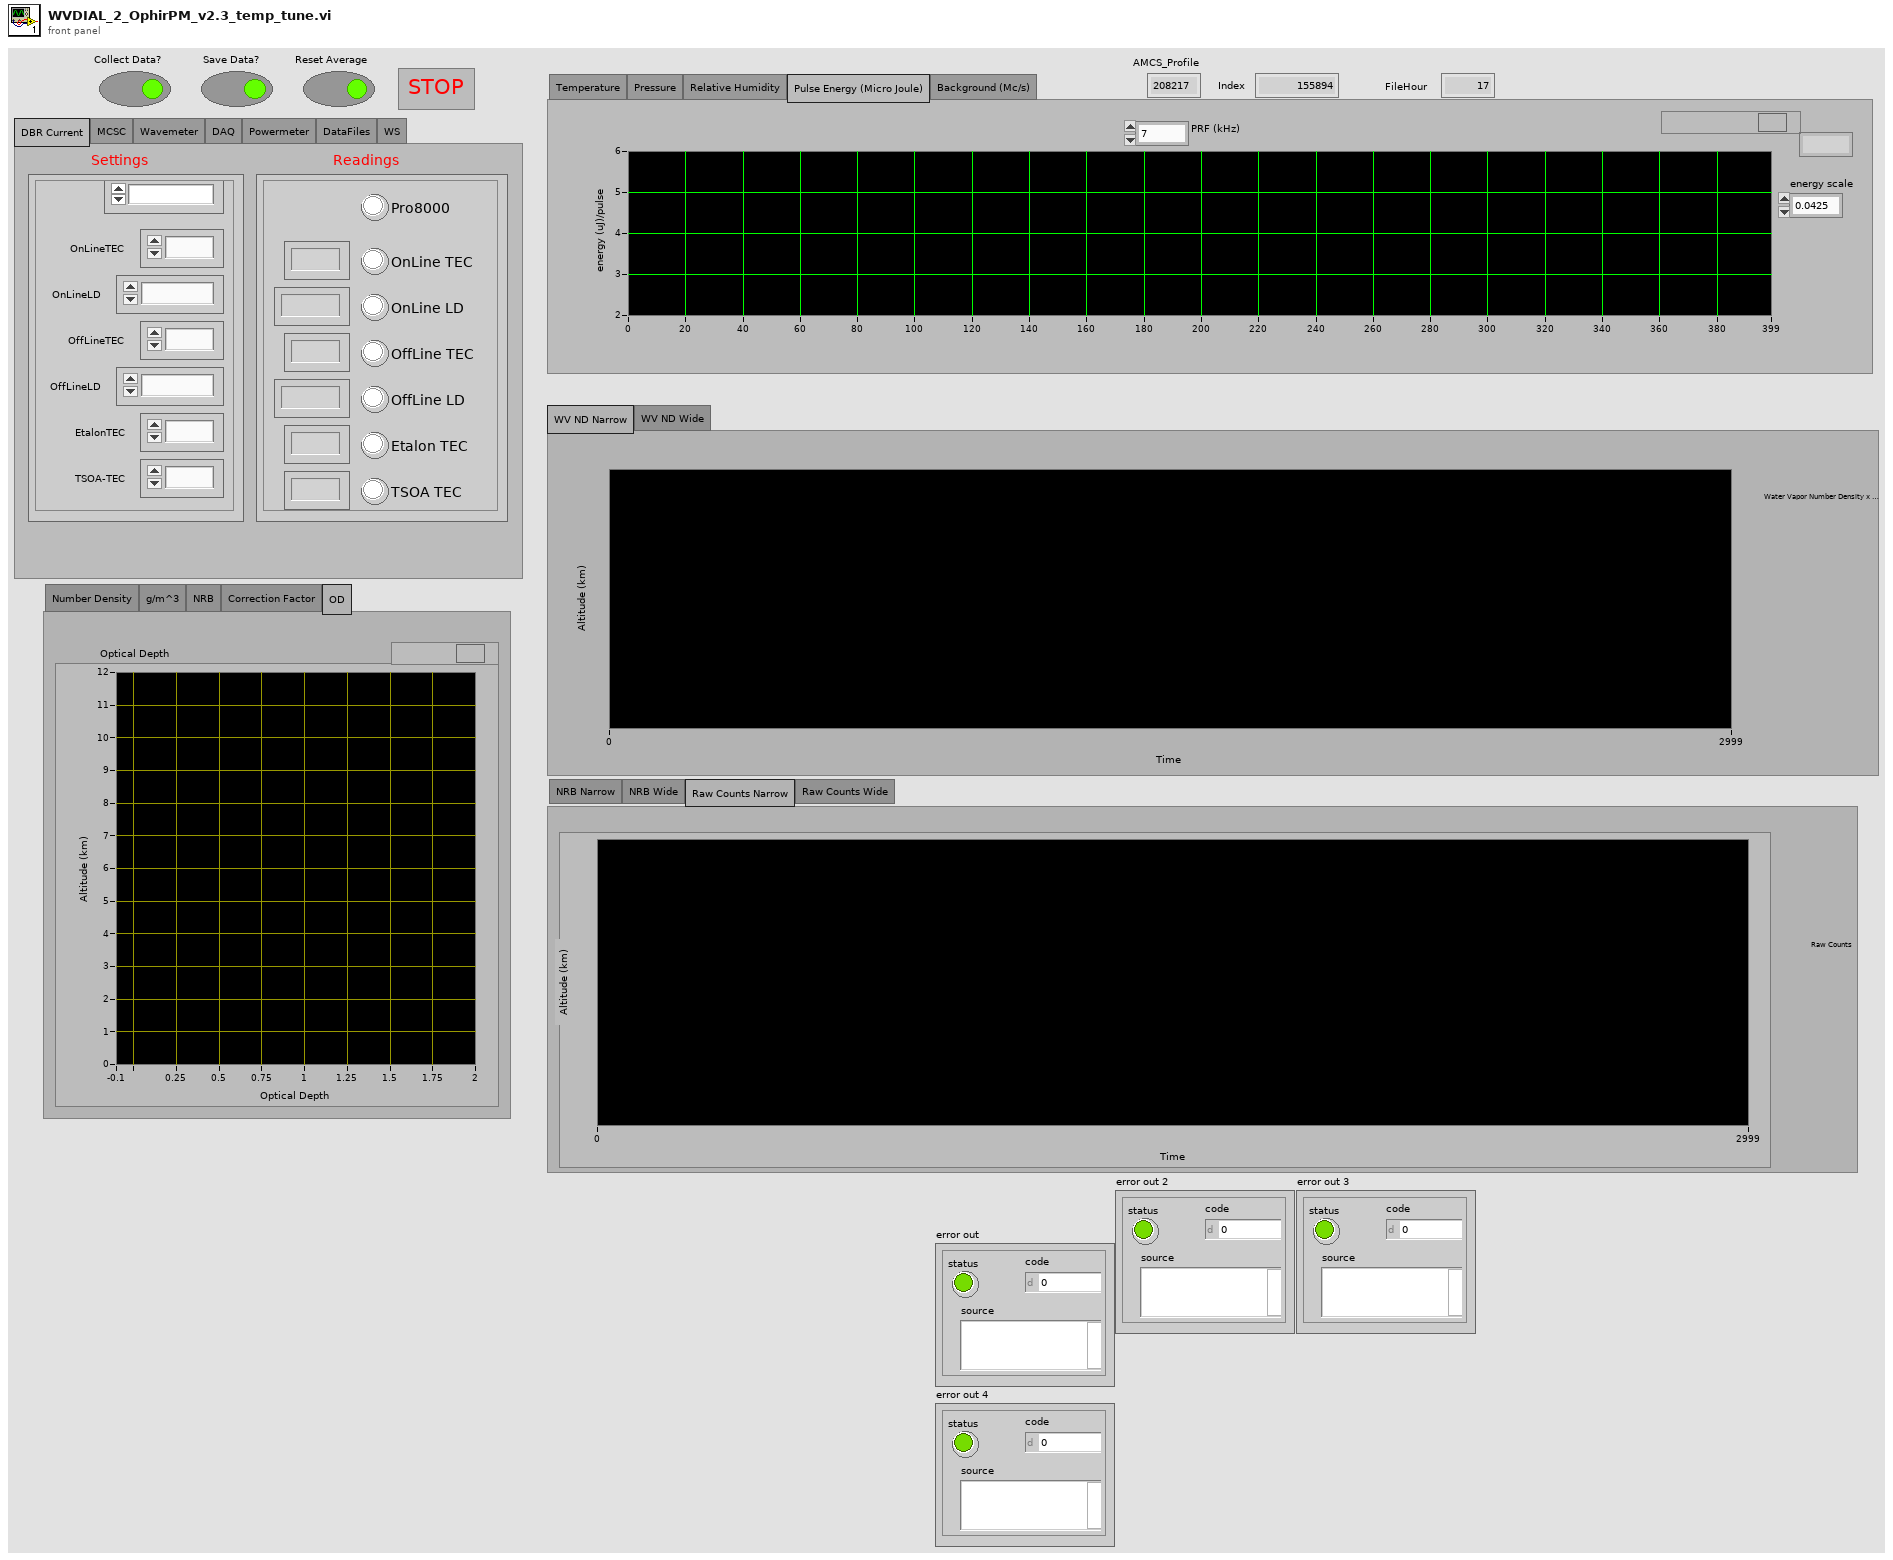
[diagram p1: front panel]
types:
  T1 = enum32{"NRB Narrow", "NRB Wide", "Raw Counts Narrow", "Raw Counts Wide"}
  T2 = enum32{"Number Density", "g/m^3", "NRB", "Correction Factor", "OD"}
  T3 = enum32{"Temperature", "Pressure", "Relative Humidity", "Pulse Energy (Micro Joule)", "Background (Mc/s)"}
  T4 = enum32{"DBR Current", "MCSC", "Wavemeter", "DAQ", "Powermeter", "DataFiles", "WS"}
  T5 = cluster{"OnLineTEC":dbl, "OnLineLD":dbl, "OffLineTEC":dbl, "OffLineLD":dbl, "EtalonTEC":dbl, "TSOA-TEC":dbl, "Pro8000":bool, "OnLine TEC":bool, "OnLine LD":bool, "OffLine TEC":bool, "OffLine LD":bool, "Etalon TEC":bool, "TSOA TEC":bool}
  T6 = cluster{"Module":enum16{"On Line TEC", "On Line LD", "Off Line TEC", "Off Line LD", "Etalon TEC", "TSOA TEC"}, "OnLineTEC":dbl, "OnLineLD":dbl, "OffLineTEC":dbl, "OffLineLD":dbl, "EtalonTEC":dbl, "TSOA-TEC":dbl}
  T7 = cluster{"Ophir-Ref":refnum<k7>, "Ophir-Device":i32, "Ophir-Channel":i32}
  T8 = cluster{"Temp C":dbl, "RelH %":dbl, "Press hPa":dbl, "AbH g/m^3":dbl}
  T9 = enum16{"Open_TL", "Close_TL", "Verify_ID", "TEC_Sensor", "SET", "READ", "ON", "OFF", "Set_Limits", "Read_Limits", "Enable_Status", "Read_Status"}
  T10 = enum16{"open", "replace", "create", "open or create", "replace or create", "replace or create with confirmation"}
  T11 = enum16{"On Line TEC", "On Line LD", "Off Line TEC", "Off Line LD", "Etalon TEC", "TSOA TEC"}
  T12 = cluster{"Temp":dbl, "RelH":dbl, "Press":dbl, "AbH":dbl}
  T13 = typedef "LVDateTimeRec.ctl" = cluster{"fractional second":dbl, "second":i32, "minute":i32, "hour":i32, "day of month":i32, "month":i32, "year":i32, "day of week":i32, "day of year":i32, "DST":i32}
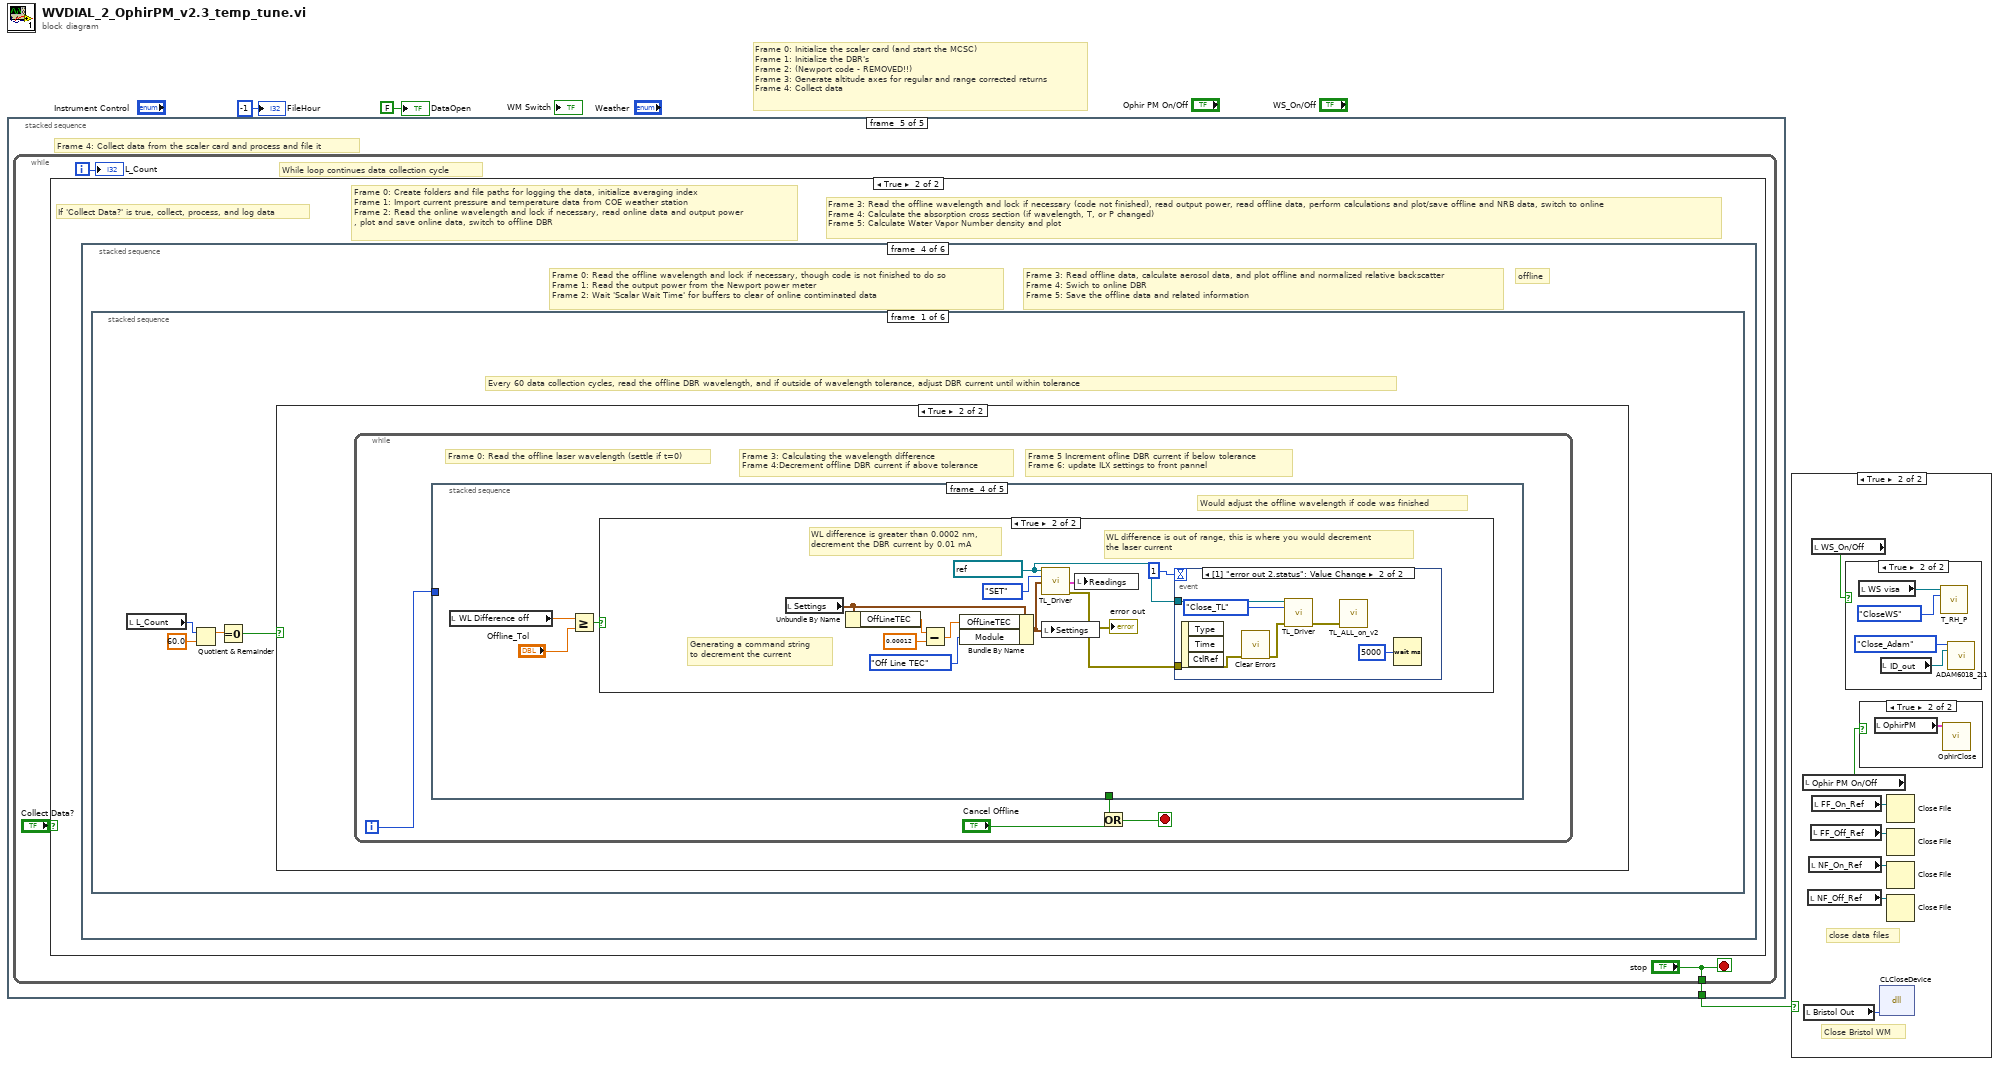
[diagram p0: block diagram]
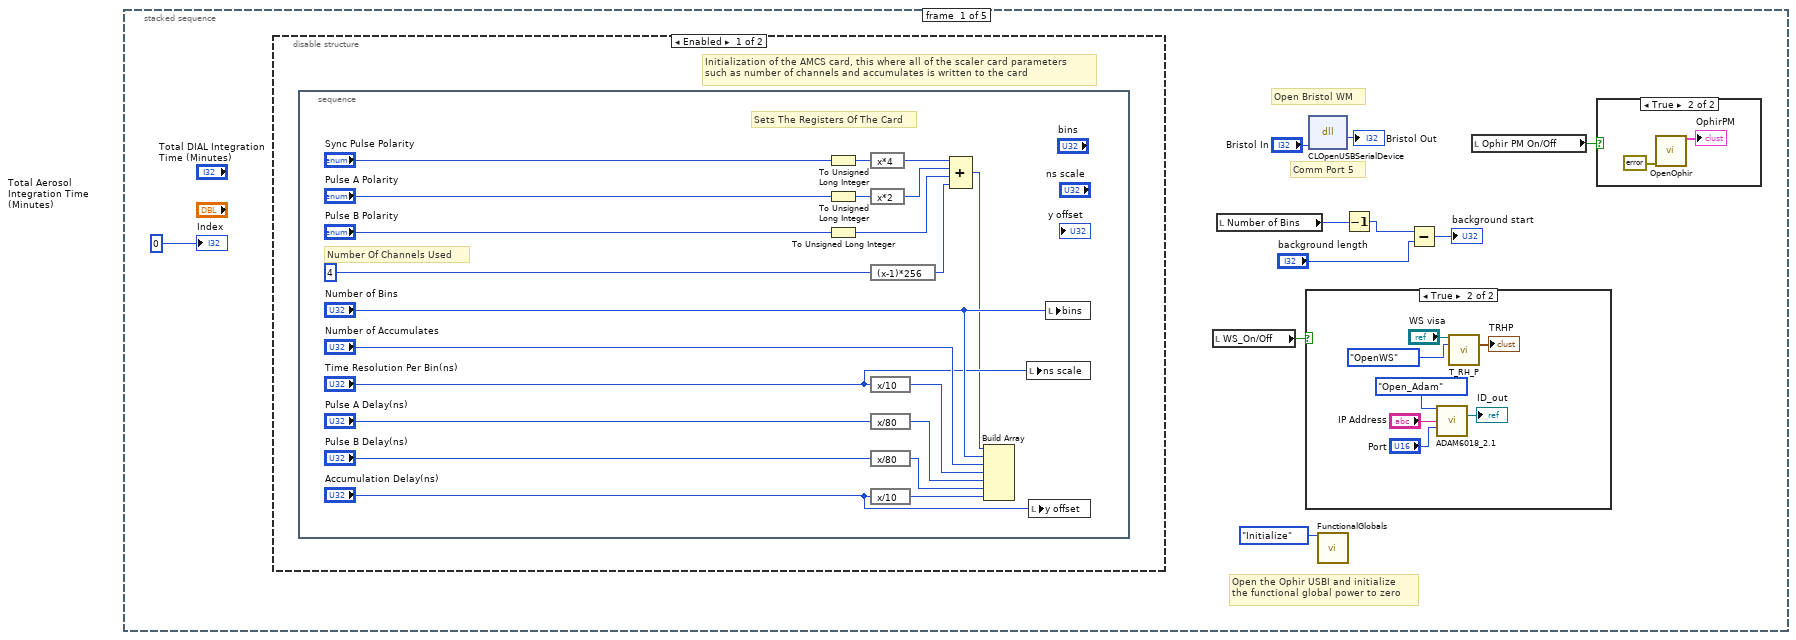
[diagram p5: hidden frame]
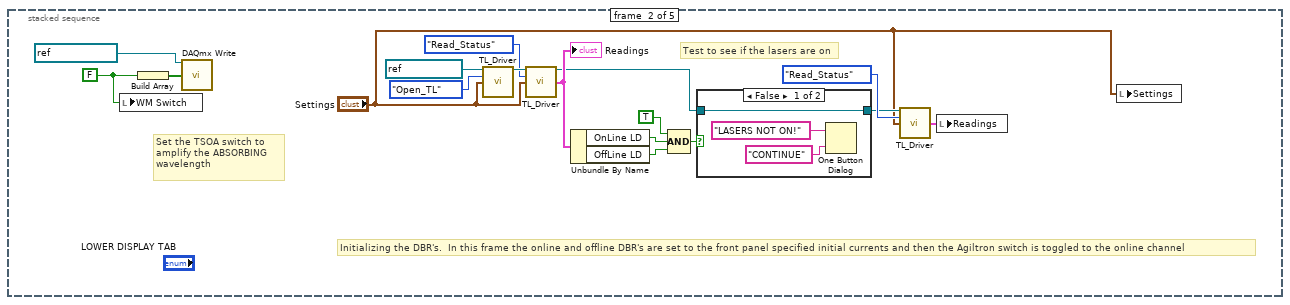
[diagram p9: hidden frame]
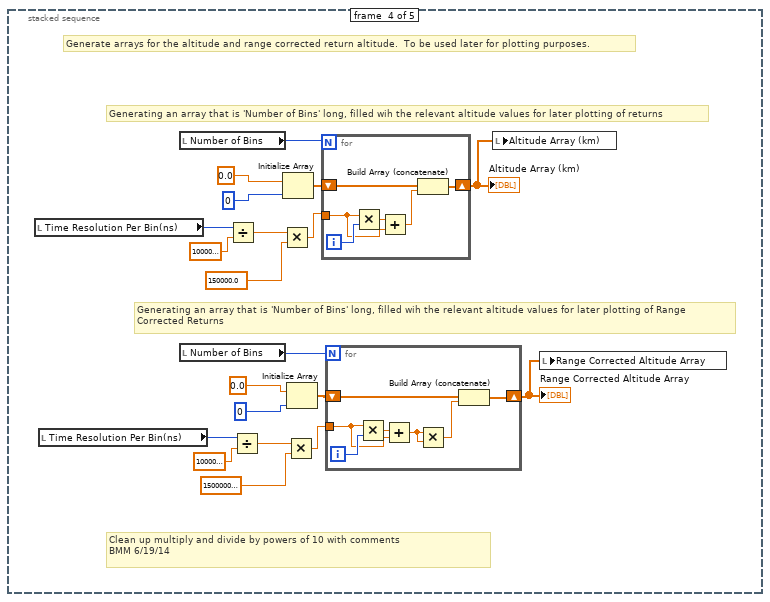
[diagram p12: hidden frame]
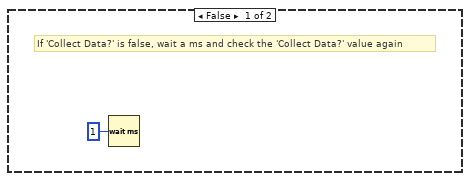
[diagram p13: hidden frame]
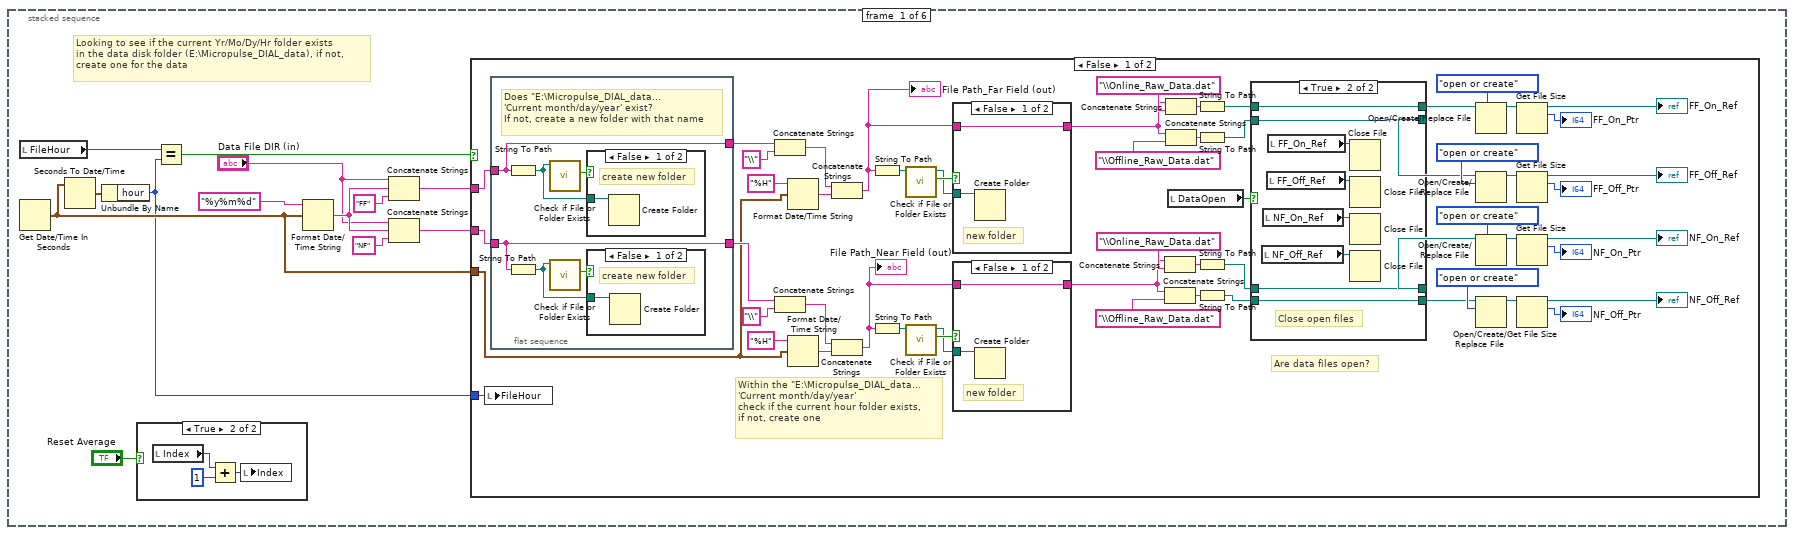
[diagram p14: hidden frame]
diagram:
  # "Frame 0: Initialize the scaler card (and start the MCSC)\nFrame 1: Initialize the DBR's\nFrame 2: (Newport code - REMOVED!!)\nFrame 3: Generate altitude axes for regular and range corrected returns\nFrame 4: Collect data"
  n1 = stacked-sequence {
    tunnel: [_ _ _ _ w98] -> w3
    frame #0 {
      # "Open the Ophir USBI and initialize\nthe functional global power to zero"
      # "Comm Port 5"
      # "Open Bristol WM"
      n2 = disable-structure shown="Enabled" {
        frame Enabled {
          # "Initialization of the AMCS card, this where all of the scaler card parameters\nsuch as number of channels and accumulates is written to the card"
          n3 = stacked-sequence {
            frame #0 {
              # "Sets The Registers Of The Card"
              # "Number Of Channels Used"
              n4 = To Unsigned Long Integer(number="Sync Pulse Polarity") -> (unsigned 32bit integer=w23:u32)
              n5 = To Unsigned Long Integer(number="Pulse A Polarity") -> (unsigned 32bit integer=w27:u32)
              n6 = To Unsigned Long Integer(number="Pulse B Polarity") -> (unsigned 32bit integer=w25:u32)
              n7 = expression code="x*4"(w23) -> (w32:u32)
              n8 = expression code="x*2"(w27) -> (w31:u32)
              n9 = expression code="(x-1)*256"(u32 4 ("Number of Channels Used")) -> (w30:u32)
              n10 = expression code="x/10"("Time Resolution Per Bin(ns)") -> (w34:u32)
              n11 = expression code="x/80"("Pulse A Delay(ns)") -> (w41:u32)
              n12 = expression code="x/80"("Pulse B Delay(ns)") -> (w43:u32)
              n13 = expression code="x/10"("Accumulation Delay(ns)") -> (w42:u32)
              n14 = Compound Arithmetic op=ADD(w32, w31, w25, w30) -> (w29:u32)
              n15 = Build Array(w29, "Number of Bins", "Number of Accumulates", w34, w41, w43, w42) -> ()  [unwired: 1 out]
              n16 = local write "ns scale"("Time Resolution Per Bin(ns)") -> ()
              n17 = local write "y offset"("Accumulation Delay(ns)") -> ()
              n18 = local write "bins"("Number of Bins") -> ()
            }
          }
        }
        frame Disabled {
        }
      }
      n19 = local read "WS_On/Off"() -> (w5:bool)
      n20 = local read "Number of Bins"() -> (w10:u32)
      n21 = case shown="True" w5 {
        frame False {
        }
        frame True {
          n22 = call "ADAM6018_2.1.vi"("ADAM6018_Command"=enum16{"Open_Adam", "Read_Adam", "Close_Adam"}."Open_Adam", "IP Address"="IP Address", "Port"="Port") -> ("ADAM_ID"=→"ID_out":refnum<k5>)  [unwired: 10 in, 2 out]
          n23 = call "T_RH_P.vi"("VISA in"="WS visa", "WS_Commands"=enum16{"OpenWS", "ReadTRHP", "CloseWS"}."OpenWS") -> ("TRHP"=→"TRHP":T12)  [unwired: 11 in, 2 out]
        }
      }
      n24 = dll-call lib="C:/H2O_DIAL/LabVIEW-2012/Bristol WM V2_31b/CLDevIface.dll" fn="CLOpenUSBSerialDevice"("commPort"="Bristol In") -> ("return type"=→"Bristol Out":i32)  [unwired: 4 in, 2 out]
      n25 = call "FunctionalGlobals.vi"("FG_Control"=enum16{"Initialize", "PowerRead", "PowerWrite"}."Initialize") -> ()  [unwired: 14 in, 1 out]
      n26 = Decrement(x=w10) -> (x-1=w9:u32)
      n27 = Subtract(x=w9, y="background length") -> (x-y=→"background start":u32)
      n28 = local read "Ophir PM On/Off"() -> (w4:bool)
      n29 = case shown="True" w4 {
        frame False {
        }
        frame True {
          n30 = call "OpenOphir.vi"("error in (no error)"=errorcluster {"status"=FALSE, "code"=0, "source"=""}) -> ("OphirPM"=→"OphirPM":T7)  [unwired: 13 in, 1 out]
        }
      }
      "Index" <- 0 ("Index")
    }
    frame #1 {
      w44 = FALSE ("Boolean")
      # "Test to see if the lasers are on"
      # "Set the TSOA switch to\namplify the ABSORBING\nwavelength"
      # "Initializing the DBR's.  In this frame the online and offline DBR's are set to the front panel specified initial currents and then the Agiltron switch is toggled to the online channel"
      n31 = local write "WM Switch"(w44) -> ()
      n32 = Build Array(w44) -> (w46:bool[])
      n33 = call-poly <vilib>:"DAQmx Write.vi"("task/channels in"=refnum<k21> "BristolWM", "data"=w46) -> ()  [unwired: 11 in, 3 out]
      n34 = call "TL_Driver.vi"("Device In"=refnum<visa-resource-name> "ThorLabs", "Commands"=T9."Open_TL", "Settings"="Settings") -> ("Device Out"=w58:refnum<visa-resource-name>)  [unwired: 9 in, 3 out]
      n35 = call "TL_Driver.vi"("Device In"=w58, "Commands"=T9."Read_Status", "Settings"="Settings") -> ("Device Out"=w55:refnum<visa-resource-name>, "Readings"=w56:T5)  [unwired: 9 in, 2 out]
      "Readings" <- w56
      n36 = Unbundle By Name(w56) -> ("OnLine LD"=w50:bool, "OffLine LD"=w51:bool)
      n37 = Compound Arithmetic op=AND(TRUE, w50, w51) -> (w49:bool)
      n38 = case shown="False" w49 {
        tunnel: w55 -> [w61 w64]
        tunnel: [w61 w64] -> w53
        frame False {
          n39 = One Button Dialog(message="LASERS NOT ON!", button name ("OK")="CONTINUE") -> ()  [unwired: 1 out]
        }
        frame True {
        }
      }
      n40 = call "TL_Driver.vi"("Device In"=w53, "Commands"=T9."Read_Status", "Settings"="Settings") -> ("Readings"=w45:T5)  [unwired: 9 in, 3 out]
      n41 = local write "Readings"(w45) -> ()
      n42 = local write "Settings"("Settings") -> ()
    }
    frame #2 {
      # "NEWPORT CODE REMOVED!!!!"
    }
    frame #3 {
      # "Clean up multiply and divide by powers of 10 with comments\nBMM 6/19/14"
      # "Generating an array that is 'Number of Bins' long, filled wih the relevant altitude values for later plotting of Range \nCorrected Returns"
      # "Generating an array that is 'Number of Bins' long, filled wih the relevant altitude values for later plotting of returns"
      # "Generate arrays for the altitude and range corrected return altitude.  To be used later for plotting purposes."
      n43 = local read "Time Resolution Per Bin(ns)"() -> (w77:u32)
      n44 = local read "Time Resolution Per Bin(ns)"() -> (w67:u32)
      n45 = local read "Number of Bins"() -> (w80:u32)
      n46 = local read "Number of Bins"() -> (w70:u32)
      n47 = Divide(x=w77, y=1000000000.0) -> (x/y=w75:dbl)
      n48 = Divide(x=w67, y=1000000000.0) -> (x/y=w65:dbl)
      n49 = Multiply(x=w75, y=150000.0) -> (x*y=w78:dbl)
      n50 = Initialize Array(0.0, 0) -> (w83:dbl[])
      n51 = Multiply(x=w65, y=150000000.0) -> (x*y=w68:dbl)
      n52 = Initialize Array(0.0, 0) -> (w73:dbl[])
      n53 = for {
        N: w80 -> [_]
        shift-right: [w96] -> w81
        shift-left: w83 -> [w97]
        tunnel: w78 -> [w93]
        i -> [w95]
        n54 = Multiply(x=w93, y=w95) -> (x*y=w94:dbl)
        n55 = Add(x=w94, y=w93) -> (x+y=w92:dbl)
        n56 = Build Array (concatenate)(w97, w92) -> (w96:dbl[])
      }
      "Altitude Array (km)" <- w81
      n57 = for {
        N: w70 -> [_]
        shift-right: [w90] -> w71
        shift-left: w73 -> [w91]
        tunnel: w68 -> [w86]
        i -> [w89]
        n58 = Multiply(x=w86, y=w89) -> (x*y=w87:dbl)
        n59 = Add(x=w87, y=w86) -> (x+y=w85:dbl)
        n60 = Multiply(x=w85, y=w85) -> (x*y=w88:dbl)
        n61 = Build Array (concatenate)(w91, w88) -> (w90:dbl[])
      }
      "Range Corrected Altitude Array" <- w71
      n62 = local write "Altitude Array (km)"(w81) -> ()
      n63 = local write "Range Corrected Altitude Array"(w71) -> ()
    }
    frame #4 {
      # "Frame 4: Collect data from the scaler card and process and file it"
      n64 = while {
        tunnel: ["stop"] -> w98
        i -> [w99]
        stop <- "stop" stop-if-true
        # "While loop continues data collection cycle"
        n65 = case shown="True" "Collect Data?" {
          frame False {
            # "If 'Collect Data?' is false, wait a ms and check the 'Collect Data?' value again"
            n66 = Wait (ms)(milliseconds to wait=u32 1) -> ()  [unwired: 1 out]
          }
          frame True {
            # "Frame 3: Read the offline wavelength and lock if necessary (code not finished), read output power, read offline data, perform calculations and plot/save offline and NRB data, switch to online\nFrame 4: Calculate the absorption cross section (if wavelength, T, or P changed)\nFrame 5: Calculate Water Vapor Number density and plot"
            # "Frame 0: Create folders and file paths for logging the data, initialize averaging index\nFrame 1: Import current pressure and temperature data from COE weather station\nFrame 2: Read the online wavelength and lock if necessary, read online data and output power\n, plot and save online data, switch to offline DBR"
            # "If 'Collect Data?' is true, collect, process, and log data"
            n67 = stacked-sequence {
              frame #0 {
                # "Looking to see if the current Yr/Mo/Dy/Hr folder exists\nin the data disk folder (E:\\Micropulse_DIAL_data), if not,\ncreate one for the data"
                n68 = local read "FileHour"() -> (w112:i32)
                n69 = Get Date/Time In Seconds() -> (seconds since 1Jan1904=w104:timestamp)
                n70 = Seconds To Date/Time(time stamp (now)=w104) -> (date time rec=w114:T13)  [unwired: 1 in]
                n71 = Unbundle By Name(w114) -> ("hour"=w103:i32)
                n72 = case shown="True" "Reset Average" {
                  frame False {
                    n73 = local write "Index"(0 ("Index")) -> ()
                  }
                  frame True {
                    n74 = local read "Index"() -> (w202:i32)
                    n75 = Add(x=w202, y=1) -> (x+y=w201:i32)
                    n76 = local write "Index"(w201) -> ()
                  }
                }
                n77 = Equal?(x=w112, y=w103) -> (x = y?=w113:bool)
                n78 = Format Date/Time String(time format string (%c)="%y%m%d", seconds (now)=w104) -> (date/time string=w108:string)  [unwired: 1 in]
                n79 = Concatenate Strings("Data File DIR (in)", w108, "FF" ("string")) -> (w110:string)
                n80 = Concatenate Strings("Data File DIR (in)", w108, "NF" ("string")) -> (w105:string)
                n81 = case shown="False" w113 {
                  tunnel: w110 -> [w172 _]
                  tunnel: w105 -> [w171 _]
                  tunnel: w104 -> [w158 _]
                  tunnel: w103 -> [w134 _]
                  frame False {
                    # "Are data files open?"
                    # "Within the \"E:\\Micropulse_DIAL_data...\n'Current month/day/year' \ncheck if the current hour folder exists,\nif not, create one"
                    n82 = local write "FileHour"(w134) -> ()
                    n83 = flat-sequence {
                      tunnel: [w192] -> w159
                      tunnel: w172 -> [w191]
                      tunnel: w171 -> [w192]
                      tunnel: [w191] -> w160
                      frame #0 {
                        # "Does \"E:\\Micropulse_DIAL_data...\n'Current month/day/year' exist?\nIf not, create a new folder with that name"
                        n84 = String To Path(string=w191) -> (path=w196:path)
                        n85 = String To Path(string=w192) -> (path=w194:path)
                        n86 = call <vilib>:"Check if File or Folder Exists.vi"("path"=w196) -> ("file or folder exists?"=w195:bool)  [unwired: 8 in, 2 out]
                        n87 = call <vilib>:"Check if File or Folder Exists.vi"("path"=w194) -> ("file or folder exists?"=w193:bool)  [unwired: 8 in, 2 out]
                        n88 = case shown="False" w195 {
                          tunnel: w196 -> [w198 _]
                          frame False {
                            # "create new folder"
                            n89 = Create Folder(path (use dialog)=w198) -> ()  [unwired: 2 in, 3 out]
                          }
                          frame True {
                            # "Folder exists\ndo nothing"
                          }
                        }
                        n90 = case shown="False" w193 {
                          tunnel: w194 -> [w197 _]
                          frame False {
                            # "create new folder"
                            n91 = Create Folder(path (use dialog)=w197) -> ()  [unwired: 2 in, 3 out]
                          }
                          frame True {
                            # "Folder exists\ndo nothing"
                          }
                        }
                      }
                    }
                    n92 = Concatenate Strings(w160, "\\" ("string")) -> (w167:string)
                    n93 = Concatenate Strings(w159, "\\" ("string")) -> (w162:string)
                    n94 = Format Date/Time String(time format string (%c)="%H", seconds (now)=w158) -> (date/time string=w170:string)  [unwired: 1 in]
                    n95 = Format Date/Time String(time format string (%c)="%H", seconds (now)=w158) -> (date/time string=w165:string)  [unwired: 1 in]
                    n96 = Concatenate Strings(w167, w170) -> (w130:string)
                    "File Path_Far Field (out)" <- w130
                    n97 = Concatenate Strings(w162, w165) -> (w131:string)
                    "File Path_Near Field (out)" <- w131
                    n98 = String To Path(string=w130) -> (path=w168:path)
                    n99 = String To Path(string=w131) -> (path=w163:path)
                    n100 = call <vilib>:"Check if File or Folder Exists.vi"("path"=w168) -> ("file or folder exists?"=w157:bool, "dup path"=w155:path)  [unwired: 8 in, 1 out]
                    n101 = call <vilib>:"Check if File or Folder Exists.vi"("path"=w163) -> ("file or folder exists?"=w156:bool, "dup path"=w154:path)  [unwired: 8 in, 1 out]
                    n102 = case shown="False" w157 {
                      tunnel: w155 -> [w189 _]
                      tunnel: w130 -> [w188 w190]
                      tunnel: [w188 w190] -> w128
                      frame False {
                        # "new folder"
                        n103 = Create Folder(path (use dialog)=w189) -> ()  [unwired: 2 in, 3 out]
                      }
                      frame True {
                        # "Folder exists\ndo nothing"
                      }
                    }
                    n104 = case shown="False" w156 {
                      tunnel: w154 -> [w186 _]
                      tunnel: w131 -> [w185 w187]
                      tunnel: [w185 w187] -> w129
                      frame False {
                        # "new folder"
                        n105 = Create Folder(path (use dialog)=w186) -> ()  [unwired: 2 in, 3 out]
                      }
                      frame True {
                        # "Folder exists\ndo nothing"
                      }
                    }
                    n106 = Concatenate Strings(w129, "\\Online_Raw_Data.dat" ("string")) -> (w148:string)
                    n107 = Concatenate Strings(w129, "\\Offline_Raw_Data.dat" ("string")) -> (w147:string)
                    n108 = Concatenate Strings(w128, "\\Online_Raw_Data.dat" ("string")) -> (w153:string)
                    n109 = Concatenate Strings(w128, "\\Offline_Raw_Data.dat" ("string")) -> (w152:string)
                    n110 = local read "DataOpen"() -> (w145:bool)
                    n111 = String To Path(string=w153) -> (path=w144:path)
                    n112 = String To Path(string=w152) -> (path=w143:path)
                    n113 = String To Path(string=w148) -> (path=w142:path)
                    n114 = String To Path(string=w147) -> (path=w141:path)
                    n115 = case shown="True" w145 {
                      tunnel: w144 -> [w176 w180]
                      tunnel: [w176 w180] -> w138
                      tunnel: w143 -> [w175 w179]
                      tunnel: [w175 w179] -> w137
                      tunnel: w142 -> [w174 w178]
                      tunnel: [w174 w178] -> w136
                      tunnel: [w173 w177] -> w135
                      tunnel: w141 -> [w173 w177]
                      frame False {
                        # "No files open\ndo nothing"
                      }
                      frame True {
                        # "Close open files"
                        n116 = local read "NF_Off_Ref"() -> (w182:refnum<file>)
                        n117 = local read "NF_On_Ref"() -> (w181:refnum<file>)
                        n118 = local read "FF_Off_Ref"() -> (w184:refnum<file>)
                        n119 = local read "FF_On_Ref"() -> (w183:refnum<file>)
                        n120 = Close File(refnum=w183) -> ()  [unwired: 1 in, 2 out]
                        n121 = Close File(refnum=w184) -> ()  [unwired: 1 in, 2 out]
                        n122 = Close File(refnum=w181) -> ()  [unwired: 1 in, 2 out]
                        n123 = Close File(refnum=w182) -> ()  [unwired: 1 in, 2 out]
                      }
                    }
                    n124 = Open/Create/Replace File(file path (use dialog)=w138, operation (0:open)=T10."open or create") -> (refnum out=w124:refnum<file>)  [unwired: 4 in, 2 out]
                    n125 = Open/Create/Replace File(file path (use dialog)=w137, operation (0:open)=T10."open or create") -> (refnum out=w125:refnum<file>)  [unwired: 4 in, 2 out]
                    n126 = Open/Create/Replace File(file path (use dialog)=w136, operation (0:open)=T10."open or create") -> (refnum out=w126:refnum<file>)  [unwired: 4 in, 2 out]
                    n127 = Open/Create/Replace File(file path (use dialog)=w135, operation (0:open)=T10."open or create") -> (refnum out=w127:refnum<file>)  [unwired: 4 in, 2 out]
                    n128 = Get File Size(file=w124) -> (refnum out=→"FF_On_Ref":refnum<file>, size (in bytes)=→"FF_On_Ptr":i64)  [unwired: 1 in, 1 out]
                    n129 = Get File Size(file=w125) -> (refnum out=→"FF_Off_Ref":refnum<file>, size (in bytes)=→"FF_Off_Ptr":i64)  [unwired: 1 in, 1 out]
                    n130 = Get File Size(file=w126) -> (refnum out=→"NF_On_Ref":refnum<file>, size (in bytes)=→"NF_On_Ptr":i64)  [unwired: 1 in, 1 out]
                    n131 = Get File Size(file=w127) -> (refnum out=→"NF_Off_Ref":refnum<file>, size (in bytes)=→"NF_Off_Ptr":i64)  [unwired: 1 in, 1 out]
                  }
                  frame True {
                    # "Don't need to do anything!"
                  }
                }
              }
              frame #1 {
                # "Writing and plotting retrieved\nweather parameters"
                # "Matlab script goes online and retrieves most recent press, temp, and relative humidity data \nfrom the weather station on the roof of Cobleigh"
                # "Importing the current weather conditions from the COE weather station"
                n132 = disable-structure shown="Disabled" {
                  frame Disabled {
                    n133 = script code="%try\n%s=urlread('http://www.coe.montana.edu/ee/weather/mostCurrentCSV.php');\n%amin=textscan(s,'%s %s %s %s %s %s %s %s %s %s %s %s %s');\n%data=amin{1}{2};\n%[test remain]=strtok(data,',');\n%remain=str2num(remain);\n%press=remain(3)./1000;\n%temp=remain(5);\n%RH=remain(7);\n%catch\npress=.850;\ntemp=20;\nRH=40;\n%end"() -> ()  [unwired: 1 in, 4 out]
                  }
                  frame Enabled {
                  }
                }
                n134 = local read "WS_On/Off"() -> (w203:bool)
                n135 = case shown="True" w203 {
                  frame False {
                  }
                  frame True {
                    n136 = disable-structure shown="Disabled" {
                      frame Disabled {
                        n137 = call "ADAM6018.vi"("Remote IP Address 2"="ADAM6018 IP") -> ()  [unwired: 10 in, 1 out]
                      }
                      frame Enabled {
                      }
                    }
                    n138 = local read "WS visa"() -> (w213:refnum<visa-resource-name>)
                    n139 = call "T_RH_P.vi"("VISA in"=w213, "WS_Commands"=enum16{"OpenWS", "ReadTRHP", "CloseWS"}."ReadTRHP") -> ("TRHP"=w208:T12)  [unwired: 11 in, 2 out]
                    n140 = local read "ID_out"() -> (w206:refnum<k5>)
                    n141 = Unbundle By Name(w208) -> ("Temp"=→"Temperature (C)":dbl, "RelH"=→"Relative Humdity (%)":dbl, "Press"=→"Pressure (mb)":dbl)
                    n142 = call "ADAM6018_2.1.vi"("ADAM6018_Command"=enum16{"Open_Adam", "Read_Adam", "Close_Adam"}."Read_Adam", "ID_in"=w206) -> ("Temps"=w207:sgl[])  [unwired: 11 in, 2 out]
                    n143 = local write "TRHP"(w208) -> ()
                    n144 = Index Array(array=w207) -> (element #1=→"T_bench":sgl)  [unwired: 8 in, 7 out]
                  }
                }
              }
              frame #2 {
                # "Frame 3: Read, process, and plot online data\nFrame 4: Switch to the offline DBR seed\nFrame 5: Write the data to the folders from Frame 0 of outter sequence"
                # "Frame 0: Read the online wavelength and adjust to locking tolerance if out of range\nFrame 1: Read the output power from the Newport meter, calculate and plot the output pulse energy\nFrame 2: Wait 'Scalar Wait Time' for buffer to clear other wavelength data"
                # "Online"
                n145 = stacked-sequence {
                  frame #0 {
                    # "Read the online wavelength and continue adjusting the online DBR if outside the wavelength tolerance\nuntil it is within tolerance"
                    n146 = while {
                      i -> [w218]
                      stop <- w216 stop-if-true
                      # "Frame 2: Decrement DBR current if above tolerance\nFrame 3: Increment DBR current if below tolerance"
                      # "Frame 0: Read the current wavelength from the wavemeter\nFrame 1: Calculate the difference between desired and actual wavelength"
                      # "Continue reading and adjusting online DBR current until within locking tolerance"
                      n147 = stacked-sequence {
                        tunnel: w218 -> [w220 _ _ _ _]
                        tunnel: [_ _ w227 _ _] -> w217
                        frame #0 {
                          n148 = Equal To 0?(x=w220) -> (x = 0?=w219:bool)
                          n149 = case shown="True" w219 {
                            frame False {
                            }
                            frame True {
                              w221 = FALSE ("Boolean")
                              # "SWITCH to ABSORBING"
                              n150 = Build Array(w221) -> (w222:bool[])
                              n151 = local write "WM Switch"(w221) -> ()
                              n152 = call-poly <vilib>:"DAQmx Write.vi"("task/channels in"=refnum<k21> "BristolWM", "data"=w222) -> ()  [unwired: 11 in, 3 out]
                            }
                          }
                        }
                        frame #1 {
                          # "Read Bristol WM"
                          n153 = local read "Bristol Out"() -> (w224:i32)
                          n154 = dll-call lib="C:/H2O_DIAL/LabVIEW-2012/Bristol WM V2_31b/CLDevIface.dll" fn="CLGetLambdaReading"("devHandle"=w224) -> ("return type"=→"Lambda On Read (nm)":dbl)  [unwired: 4 in, 2 out]
                        }
                        frame #2 {
                          # "If WL difference is within tolerance, stop looping, and illuminate 'Wavelength Lock Online' indicator"
                          # "Calculating the difference between the actual and desired online wavelength"
                          n155 = local read "Lambda On Read (nm)"() -> (w234:dbl)
                          n156 = local read "Online_Tol"() -> (w231:dbl)
                          n157 = Subtract(x=w234, y="Lambda On Set (nm)") -> (x-y=w226:dbl)
                          "WL Difference" <- w226
                          n158 = Multiply(x=-1.0, y=w231) -> (x*y=w232:dbl)
                          n159 = Greater?(x=w226, y=w232) -> (0:w228:bool)
                          n160 = Less?(x=w226, y=w231) -> (x < y?=w229:bool)
                          n161 = And(x=w228, y=w229) -> (x .and. y?=w227:bool)
                          "Wavelength Lock Online" <- w227
                        }
                        frame #3 {
                          # "If the wavelength difference is greater that 0.0002 nm, decrement the \nDBR current by 0.01 mA"
                          n162 = local read "WL Difference"() -> (w237:dbl)
                          n163 = Greater Or Equal?(x=w237, y="Online_Tol") -> (x >= y?=w235:bool)
                          n164 = case shown="True" w235 {
                            frame False {
                              # "Wavelength difference is not greater than 0.0002 nm, do nothing"
                            }
                            frame True {
                              # "Generating a command string\nto decrement the current"
                              # "WL difference is greater than 0.0002 nm,\ndecrement the DBR current by 0.01 mA"
                              n165 = local read "Settings"() -> (w245:T6)
                              n166 = Unbundle By Name(w245) -> ("OnLineTEC"=w247:dbl)
                              n167 = Subtract(x=w247, y=0.00012) -> (x-y=w248:dbl)
                              n168 = Bundle By Name(cluster=w245, "OnLineTEC"=w248, "Module"=T11."On Line TEC") -> (w243:T6)
                              n169 = call "TL_Driver.vi"("Device In"=refnum<visa-resource-name> "ThorLabs", "Commands"=T9."SET", "Settings"=w243) -> ("Device Out"=w238:refnum<visa-resource-name>, "Readings"=w241:T5, "error out"=w240:errorcluster)  [unwired: 9 in, 1 out]
                              "error out 3" <- w240
                              n170 = local write "Settings"(w243) -> ()
                              n171 = local write "Readings"(w241) -> ()
                              n172 = event shown="[1] \"error out 3.status\": Value Change" {
                                selector: _ -> [_ _]
                                dyn-events: _ -> [_ _]
                                timeout: 1 -> [_ _]
                                tunnel: w238 -> [_ w255]
                                tunnel: w240 -> [_ w254]
                                event Timeout {
                                n173 = event-data() -> ()  [unwired: 1 in, 2 out]
                                }
                                event "error out 3.status": Value Change {
                                n174 = event-data() -> ()  [unwired: 1 in, 4 out]
                                n175 = call <vilib>:"Clear Errors.vi"("error in (no error)"=w254) -> ("error out"=w251:errorcluster)  [unwired: 6 in]
                                n176 = call "TL_Driver.vi"("Device In"=w255, "Commands"=T9."Close_TL", "error in"=w251) -> ("error out"=w250:errorcluster)  [unwired: 9 in, 3 out]
                                n177 = call "TL_ALL_on_v2.vi"("error in"=w250) -> ()  [unwired: 11 in]
                                n178 = Wait (ms)(milliseconds to wait=u32 5000) -> ()  [unwired: 1 out]
                                }
                              }
                            }
                          }
                        }
                        frame #4 {
                          # "If the wavelength difference is less that 0.0002 nm, increment the \nDBR current by 0.01 mA"
                          n179 = local read "WL Difference"() -> (w260:dbl)
                          n180 = local read "Online_Tol"() -> (w258:dbl)
                          n181 = Multiply(x=-1.0, y=w258) -> (x*y=w256:dbl)
                          n182 = Less Or Equal?(x=w260, y=w256) -> (x <= y?=w259:bool)
                          n183 = case shown="True" w259 {
                            frame False {
                              # "WL difference is no <= to -0.0002 nm, do nothing"
                            }
                            frame True {
                              w263 = refnum<visa-resource-name> "ThorLabs" ("Device In")
                              # "WL difference is < -0.0002,\nincrement the DBR current by 0.01 mA"
                              # "Generating a command string\nto decrement the current"
                              n184 = local read "Settings"() -> (w267:T6)
                              n185 = Unbundle By Name(w267) -> ("OnLineTEC"=w269:dbl)
                              n186 = Add(x=w269, y=0.00012) -> (x+y=w270:dbl)
                              n187 = Bundle By Name(cluster=w267, "OnLineTEC"=w270, "Module"=T11."On Line TEC") -> (w265:T6)
                              n188 = call "TL_Driver.vi"("Device In"=w263, "Commands"=T9."SET", "Settings"=w265) -> ("Readings"=w264:T5, "error out"=w262:errorcluster)  [unwired: 9 in, 2 out]
                              "error out 4" <- w262
                              n189 = local write "Settings"(w265) -> ()
                              n190 = local write "Readings"(w264) -> ()
                              n191 = event shown="[1] \"error out 4.status\": Value Change" {
                                selector: _ -> [_ _]
                                dyn-events: _ -> [_ _]
                                timeout: 1 -> [_ _]
                                tunnel: w263 -> [_ w277]
                                tunnel: w262 -> [_ w276]
                                event Timeout {
                                n192 = event-data() -> ()  [unwired: 1 in, 2 out]
                                }
                                event "error out 4.status": Value Change {
                                n193 = event-data() -> ()  [unwired: 1 in, 4 out]
                                n194 = call <vilib>:"Clear Errors.vi"("error in (no error)"=w276) -> ("error out"=w273:errorcluster)  [unwired: 6 in]
                                n195 = call "TL_Driver.vi"("Device In"=w277, "Commands"=T9."Close_TL", "error in"=w273) -> ("error out"=w272:errorcluster)  [unwired: 9 in, 3 out]
                                n196 = call "TL_ALL_on_v2.vi"("error in"=w272) -> ()  [unwired: 11 in]
                                n197 = Wait (ms)(milliseconds to wait=u32 5000) -> ()  [unwired: 1 out]
                                }
                              }
                            }
                          }
                        }
                      }
                      n198 = Or(x=w217, y="Cancel online") -> (x .or. y?=w216:bool)
                    }
                  }
                  frame #1 {
                    # "Reading the output power of the laser transmitter from the Ophir power meter, once read, convert to corresponding pulse energy and plot"
                    n199 = local read "Ophir PM On/Off"() -> (w278:bool)
                    n200 = case shown="True" w278 {
                      frame False {
                      }
                      frame True {
                        # "Plotting the online and offling pulse energies"
                        # "Converting to pulse energy, assumes 5 percent pickoff"
                        n201 = local read "OphirPM"() -> (w283:T7)
                        n202 = call "OphirRead.vi"("OphirPM"=w283) -> ("Power (W)"=w279:dbl, "Ophir Samples"=→"Ophir Samples":i32)  [unwired: 12 in, 1 out]
                        "Average Diode Power" <- w279
                        n203 = Multiply(x=w279, y=1000.0) -> (x*y=w287:dbl)
                        n204 = Divide(x=w287, y="energy scale") -> (x/y=w285:dbl)
                        n205 = Divide(x=w285, y="PRF (kHz)") -> (x/y=w280:dbl)
                        n206 = Bundle(w280) -> (→"Pulse Energy (Micro Joule)":cluster{dbl})  [unwired: 1 in]
                      }
                    }
                  }
                  frame #2 {
                    # "Wait 'Scalar Wait Time' for the next available batch of scalar card data"
                    n207 = local read "AMCS_Profile"() -> (w289:i32)
                    n208 = disable-structure shown="Disabled" {
                      frame Disabled {
                        # "Waiting 'Scalar Wait Time'"
                        n209 = Wait (ms)(milliseconds to wait="Scalar Wait Time (disabled)") -> ()  [unwired: 1 out]
                      }
                      frame Enabled {
                      }
                    }
                    n210 = while {
                      tunnel: [w296] -> w290
                      tunnel: [w292] -> _
                      tunnel: w289 -> [w292]
                      stop <- w294 stop-if-true
                      n211 = global read "AMCS_Data.vi" "AMCS_Profile"() -> (w296:i32)
                      n212 = Wait (ms)(milliseconds to wait=u32 10) -> ()  [unwired: 1 out]
                      n213 = Equal?(x=w296, y=w292) -> (x = y?=w295:bool)
                      n214 = case shown="False" w295 {
                        tunnel: [TRUE FALSE] -> w294
                        frame False {
                        }
                        frame True {
                        }
                      }
                    }
                    "AMCS_Profile" <- w290
                  }
                  frame #3 {
                    # "convert time per range bin to meters\nand calculate smoothed bins using\nsmoothing range"
                    # "Plotting online cross section and smoothed online data"
                    # "Calculate the bin by bin mean of the data"
                    # "Collect 'Integration Period (Seconds)' number\nof scalar data"
                    # "Reading, processing, and plotting the online data"
                    n215 = local read "Data Reads (number of loops)"() -> (w324:i32)
                    n216 = for {
                      N: w324 -> [_]
                      tunnel: [w344] -> w336 mode=indexing
                      tunnel: [w345] -> w316 mode=indexing
                      # "Scalar Data is retrieved from Global \nVariable that scaler.vi is writing to,"
                      n217 = disable-structure shown="Disabled" {
                        frame Disabled {
                          n218 = global read "Scalar_Data.vi" "Scalar Data  3"() -> ()  [unwired: 1 out]
                          n219 = global read "Scalar_Data.vi" "Scalar Data"() -> ()  [unwired: 1 out]
                        }
                        frame Enabled {
                        }
                      }
                      n220 = global read "AMCS_Data.vi" "AMCS_Data"() -> (w348:u16[][])
                      n221 = Index Array(array=w348, index (row) #1=0 ("index (row)"), index (row) #2=2 ("index (row)")) -> (element #1=w344:u16[], element #2=w345:u16[])  [unwired: 2 in]
                    }
                    n222 = Transpose 2D Array(2D array=w336) -> (transposed array=w340:u16[][])
                    n223 = Transpose 2D Array(2D array=w316) -> (transposed array=w322:u16[][])
                    n224 = for {
                      tunnel: w340 -> [w350] mode=indexing
                      tunnel: [w349] -> w341 mode=indexing
                      n225 = call-poly <vilib>:"Mean.vi"("X"=w350) -> ("mean"=w349:dbl)  [unwired: 1 out]
                    }
                    n226 = for {
                      tunnel: w322 -> [w343] mode=indexing
                      tunnel: [w342] -> w323 mode=indexing
                      n227 = call-poly <vilib>:"Mean.vi"("X"=w343) -> ("mean"=w342:dbl)  [unwired: 1 out]
                    }
                    n228 = local read "bins"() -> (w315:u32)
                    n229 = Array Subset(array=w341, index=1 ("dimension size"), length=w315) -> (w328:dbl[])
                    n230 = Array Subset(array=w323, index=1 ("dimension size"), length=w315) -> (w320:dbl[])
                    n231 = local read "background length"() -> (w305:i32)
                    n232 = local read "background start"() -> (w306:u32)
                    n233 = Array Size(array=w328) -> (size(s)=w325:i32)
                    n234 = Array Size(array=w320) -> (size(s)=w317:i32)
                    n235 = Initialize Array(1.0 ("element"), w325) -> (w327:dbl[])
                    n236 = Initialize Array(1.0 ("element"), w317) -> (w319:dbl[])
                    n237 = Multiply(x=w328, y=w327) -> (x*y=w329:dbl[])
                    "On-Line Bin Readings" <- w329
                    n238 = Multiply(x=w320, y=w319) -> (x*y=w309:dbl[])
                    "On-Line Bin Readings 2" <- w309
                    n239 = local read "Total DIAL Integration Time (Minutes)"() -> (w332:i32)
                    n240 = local read "Time Resolution Per Bin(ns)"() -> (w301:u32)
                    n241 = Array Subset(array=w329, index=w306, length=w305) -> (w338:dbl[])
                    n242 = Array Subset(array=w309, index=w306, length=w305) -> (w311:dbl[])
                    n243 = call-poly <vilib>:"Mean.vi"("X"=w338) -> ("mean"=w337:dbl)  [unwired: 1 out]
                    n244 = call-poly <vilib>:"Mean.vi"("X"=w311) -> ("mean"=w312:dbl)  [unwired: 1 out]
                    n245 = Divide(x=w332, y=w324) -> (x/y=w330:dbl)
                    n246 = local read "Index"() -> (w310:i32)
                    n247 = Subtract(x=w329, y=w337) -> (x-y=w334:dbl[])
                    n248 = Subtract(x=w309, y=w312) -> (x-y=w313:dbl[])
                    n249 = To Double Precision Float(number=w301) -> (double precision float=w302:dbl)
                    n250 = Multiply(x=w330, y=60.0) -> (x*y=w307:dbl)
                    n251 = Multiply(x=w302, y=0.15) -> (x*y=w304:dbl)
                    n252 = call "Ring Buffer Online Far.vi"("Index"=w310, "Profiles to Average"=w307, "Input Array"=w334) -> ("AvgArray"=w333:dbl[])  [unwired: 7 in, 1 out]
                    n253 = call "Ring Buffer Online Near.vi"("Index"=w310, "Profiles to Average"=w307, "Input Array"=w313) -> ("AvgArray"=w314:dbl[])  [unwired: 7 in, 1 out]
                    n254 = Divide(x="Smoothing Range", y=w304) -> (x/y=w299:dbl)
                    "Smoothed Bins" <- w299
                    n255 = call "Smooth Arrray.vi"("smooth size"=w299, "Raw Array"=w333) -> ("Smoothed Array"=→"On-Line  Smoothed":dbl[])  [unwired: 9 in]
                    n256 = call "Smooth Arrray.vi"("smooth size"=w299, "Raw Array"=w314) -> ("Smoothed Array"=→"On-Line Smoothed 2":dbl[])  [unwired: 9 in]
                    n257 = disable-structure shown="Disabled" {
                      frame Disabled {
                        n258 = script code="format long;\ncounts=sum(Online);\nif counts >=0.5e6\ntime=time;\nelse\ntime=time\nend"() -> ()  [unwired: 3 in, 2 out]
                      }
                      frame Enabled {
                      }
                    }
                  }
                  frame #4 {
                    # "CODE REMOVED!!"
                    # "Toggling the Agiltron switch to the offline DBR seed laser"
                  }
                  frame #5 {
                    # "Save the recently collected online data if 'Save Data?' is true"
                    n259 = case shown="True" "Save Data?" {
                      frame False {
                        # "'Save Data?' is false, do nothing"
                      }
                      frame True {
                        # "'Save Data?' is true, save onfline data to the Data Disk"
                        # "Write only one copy of data at this time"
                        # "Retrieve Julian Date"
                        n260 = local read "Readings"() -> (w359:T5)
                        n261 = local read "Time Resolution Per Bin(ns)"() -> (w357:u32)
                        n262 = local read "Number of Accumulates"() -> (w355:u32)
                        n263 = local read "Number of Bins"() -> (w356:u32)
                        n264 = local write "DataOpen"(TRUE ("DataOpen")) -> ()
                        n265 = local read "Lambda On Read (nm)"() -> (w381:dbl)
                        n266 = local read "On-Line Bin Readings 2"() -> (w379:dbl[])
                        n267 = local read "On-Line Bin Readings"() -> (w383:dbl[])
                        n268 = local read "Average Diode Power"() -> (w380:dbl)
                        n269 = Unbundle By Name(w359) -> ("OnLineLD"=w358:dbl)
                        n270 = To Double Precision Float(number=w357) -> (double precision float=w354:dbl)
                        n271 = To Double Precision Float(number=w356) -> (double precision float=w353:dbl)
                        n272 = To Double Precision Float(number=w355) -> (double precision float=w352:dbl)
                        n273 = call "Julian_Date_2.vi"() -> ("Julian Date"=w382:dbl)  [unwired: 11 in]
                        n274 = Build Array (concatenate)(w382, w381, w358, w380, w354, w353, w352, w383) -> (w374:dbl[])
                        n275 = Build Array (concatenate)(w382, w381, w358, w380, w354, w353, w352, w379) -> (w364:dbl[])
                        n276 = local read "NF_On_Ref"() -> (w362:refnum<file>)
                        n277 = local read "FF_On_Ref"() -> (w378:refnum<file>)
                        n278 = local read "NF_On_Ptr"() -> (w363:i64)
                        n279 = local read "FF_On_Ptr"() -> (w377:i64)
                        n280 = Set File Position(offset (in bytes) (0)=w377, refnum=w378) -> (refnum out=w375:refnum<file>, error out=w372:errorcluster)  [unwired: 2 in]
                        n281 = Set File Position(offset (in bytes) (0)=w363, refnum=w362) -> (refnum out=w368:refnum<file>, error out=w366:errorcluster)  [unwired: 2 in]
                        n282 = Write to Binary File(file (use dialog)=w368, data=w364, error in=w366, 5:FALSE ("prepend array or string size? (T)")) -> (refnum out=w367:refnum<file>, error out=w365:errorcluster)  [unwired: 2 in, 1 out]
                        n283 = Write to Binary File(file (use dialog)=w375, data=w374, error in=w372, 5:FALSE ("prepend array or string size? (T)")) -> (refnum out=w373:refnum<file>, error out=w371:errorcluster)  [unwired: 2 in, 1 out]
                        n284 = Get File Position(4:w365, 7:w367) -> (2:w361:i64)  [unwired: 2 out]
                        n285 = Get File Position(4:w371, 7:w373) -> (2:w370:i64)  [unwired: 2 out]
                        n286 = local write "NF_On_Ptr"(w361) -> ()
                        n287 = local write "FF_On_Ptr"(w370) -> ()
                      }
                    }
                  }
                }
              }
              frame #3 {
                # "Frame 3: Read offline data, calculate aerosol data, and plot offline and normalized relative backscatter\nFrame 4: Swich to online DBR\nFrame 5: Save the offline data and related information"
                # "Frame 0: Read the offline wavelength and lock if necessary, though code is not finished to do so\nFrame 1: Read the output power from the Newport power meter\nFrame 2: Wait 'Scalar Wait Time' for buffers to clear of online contiminated data"
                # "offline"
                n288 = stacked-sequence {
                  frame #0 {
                    # "Every 60 data collection cycles, read the offline DBR wavelength, and if outside of wavelength tolerance, adjust DBR current until within tolerance"
                    n289 = local read "L_Count"() -> (w385:i32)
                    n290 = Quotient & Remainder(x=w385, y=60.0) -> (x-y*floor(x/y)=w386:dbl)  [unwired: 1 out]
                    n291 = Equal To 0?(x=w386) -> (x = 0?=w384:bool)
                    n292 = case shown="True" w384 {
                      frame False {
                      }
                      frame True {
                        n293 = while {
                          i -> [w391]
                          stop <- w389 stop-if-true
                          # "Frame 5 Increment ofline DBR current if below tolerance\nFrame 6: update ILX settings to front pannel"
                          # "Frame 3: Calculating the wavelength difference\nFrame 4:Decrement offline DBR current if above tolerance"
                          # "Frame 0: Read the offline laser wavelength (settle if t=0)"
                          n294 = stacked-sequence {
                            tunnel: w391 -> [w393 _ _ _ _]
                            tunnel: [_ _ w403 _ _] -> w390
                            frame #0 {
                              n295 = Equal To 0?(x=w393) -> (x = 0?=w392:bool)
                              n296 = case shown="True" w392 {
                                frame False {
                                }
                                frame True {
                                w394 = TRUE ("Boolean")
                                # "SWITCH to NON-ABSORBING and wait to settle"
                                n297 = Build Array(w394) -> (w399:bool[])
                                n298 = local write "WM Switch"(w394) -> ()
                                n299 = call-poly <vilib>:"DAQmx Write.vi"("task/channels in"=refnum<k21> "BristolWM", "data"=w399) -> ()  [unwired: 11 in, 3 out]
                                n300 = call "TL_Driver.vi"("Device In"=refnum<visa-resource-name> "ThorLabs", "Commands"=T9."Read_Status") -> ("Readings"=w397:T5)  [unwired: 10 in, 3 out]
                                n301 = local write "Readings"(w397) -> ()
                                n302 = Wait (ms)(milliseconds to wait=u32 3200) -> ()  [unwired: 1 out]
                                }
                              }
                            }
                            frame #1 {
                              # "Read Bristol WM"
                              n303 = local read "Bristol Out"() -> (w401:i32)
                              n304 = dll-call lib="C:/H2O_DIAL/LabVIEW-2012/Bristol WM V2_31b/CLDevIface.dll" fn="CLGetLambdaReading"("devHandle"=w401) -> ("return type"=→"Lambda Off Read (nm)":dbl)  [unwired: 4 in, 2 out]
                            }
                            frame #2 {
                              # "Once locked, stop looping and illuminate 'Wavelength Lock Offline'"
                              # "While loop continues locking process until the wavelength is within tolerance"
                              # "Calculating the difference between the actual and desired \noffline wavelength"
                              n305 = local read "Lambda Off Read (nm)"() -> (w411:dbl)
                              n306 = Subtract(x=w411, y="Lambda Off Set (nm)") -> (x-y=w404:dbl)
                              "WL Difference off" <- w404
                              n307 = local read "Offline_Tol"() -> (w408:dbl)
                              n308 = Multiply(x=-1.0, y=w408) -> (x*y=w409:dbl)
                              n309 = Greater?(x=w404, y=w409) -> (0:w405:bool)
                              n310 = Less?(x=w404, y=w408) -> (x < y?=w406:bool)
                              n311 = And(x=w405, y=w406) -> (x .and. y?=w403:bool)
                              "Wavelength Lock Offline" <- w403
                              n312 = case shown="True" w403 {
                                frame False {
                                }
                                frame True {
                                w412 = FALSE ("Boolean")
                                # "SWITCH back to ABSORBING and wait to settle"
                                n313 = Build Array(w412) -> (w414:bool[])
                                n314 = local write "WM Switch"(w412) -> ()
                                n315 = call-poly <vilib>:"DAQmx Write.vi"("task/channels in"=refnum<k21> "BristolWM", "data"=w414) -> ()  [unwired: 11 in, 3 out]
                                n316 = Wait (ms)(milliseconds to wait=u32 3200) -> ()  [unwired: 1 out]
                                }
                              }
                            }
                            frame #3 {
                              # "Would adjust the offline wavelength if code was finished"
                              n317 = local read "WL Difference off"() -> (w418:dbl)
                              n318 = Greater Or Equal?(x=w418, y="Offline_Tol") -> (x >= y?=w416:bool)
                              n319 = case shown="True" w416 {
                                frame False {
                                # "WL difference is not out of range, do nothing"
                                }
                                frame True {
                                w421 = refnum<visa-resource-name> "ThorLabs" ("Device In")
                                # "Generating a command string\nto decrement the current"
                                # "WL difference is greater than 0.0002 nm,\ndecrement the DBR current by 0.01 mA"
                                # "WL difference is out of range, this is where you would decrement\nthe laser current"
                                n320 = local read "Settings"() -> (w426:T6)
                                n321 = Unbundle By Name(w426) -> ("OffLineTEC"=w427:dbl)
                                n322 = Subtract(x=w427, y=0.00012) -> (x-y=w428:dbl)
                                n323 = Bundle By Name(cluster=w426, "OffLineTEC"=w428, "Module"=T11."Off Line TEC") -> (w425:T6)
                                n324 = call "TL_Driver.vi"("Device In"=w421, "Commands"=T9."SET", "Settings"=w425) -> ("Readings"=w422:T5, "error out"=w420:errorcluster)  [unwired: 9 in, 2 out]
                                "error out" <- w420
                                n325 = local write "Settings"(w425) -> ()
                                n326 = local write "Readings"(w422) -> ()
                                n327 = event shown="[1] \"error out 2.status\": Value Change" {
                                selector: _ -> [_ _]
                                dyn-events: _ -> [_ _]
                                timeout: 1 -> [_ _]
                                tunnel: w421 -> [_ w435]
                                tunnel: w420 -> [_ w434]
                                event Timeout {
                                n328 = event-data() -> ()  [unwired: 1 in, 2 out]
                                }
                                event "error out 2.status": Value Change {
                                n329 = event-data() -> ()  [unwired: 1 in, 3 out]
                                n330 = call <vilib>:"Clear Errors.vi"("error in (no error)"=w434) -> ("error out"=w431:errorcluster)  [unwired: 6 in]
                                n331 = call "TL_Driver.vi"("Device In"=w435, "Commands"=T9."Close_TL", "error in"=w431) -> ("error out"=w430:errorcluster)  [unwired: 9 in, 3 out]
                                n332 = call "TL_ALL_on_v2.vi"("error in"=w430) -> ()  [unwired: 11 in]
                                n333 = Wait (ms)(milliseconds to wait=u32 5000) -> ()  [unwired: 1 out]
                                }
                                }
                                }
                              }
                            }
                            frame #4 {
                              # "This is where you would increment the offline current if below tolerance"
                              n334 = local read "Offline_Tol"() -> (w437:dbl)
                              n335 = local read "WL Difference off"() -> (w440:dbl)
                              n336 = Multiply(x=-1.0, y=w437) -> (x*y=w436:dbl)
                              n337 = Less Or Equal?(x=w440, y=w436) -> (x <= y?=w439:bool)
                              n338 = case shown="True" w439 {
                                frame False {
                                # "WL difference is not outisde tolerance, do nothing"
                                }
                                frame True {
                                w443 = refnum<visa-resource-name> "ThorLabs" ("Device In")
                                # "Generating a command string\nto decrement the current"
                                # "WL difference is less than 0.0002 nm,\nincrement the DBR current by 0.01 mA"
                                # "Incrementing the current if below tolerance"
                                n339 = local read "Settings"() -> (w447:T6)
                                n340 = Unbundle By Name(w447) -> ("OffLineTEC"=w449:dbl)
                                n341 = Add(x=w449, y=0.00012) -> (x+y=w450:dbl)
                                n342 = Bundle By Name(cluster=w447, "OffLineTEC"=w450, "Module"=T11."Off Line TEC") -> (w448:T6)
                                n343 = call "TL_Driver.vi"("Device In"=w443, "Commands"=T9."SET", "Settings"=w448) -> ("Readings"=w444:T5, "error out"=w442:errorcluster)  [unwired: 9 in, 2 out]
                                "error out 2" <- w442
                                n344 = local write "Settings"(w448) -> ()
                                n345 = local write "Readings"(w444) -> ()
                                n346 = event shown="[1] \"error out.status\": Value Change" {
                                selector: _ -> [_ _]
                                dyn-events: _ -> [_ _]
                                timeout: 1 -> [_ _]
                                tunnel: w443 -> [_ w457]
                                tunnel: w442 -> [_ w456]
                                event Timeout {
                                n347 = event-data() -> ()  [unwired: 1 in, 2 out]
                                }
                                event "error out.status": Value Change {
                                n348 = event-data() -> ()  [unwired: 1 in, 4 out]
                                n349 = call <vilib>:"Clear Errors.vi"("error in (no error)"=w456) -> ("error out"=w453:errorcluster)  [unwired: 6 in]
                                n350 = call "TL_Driver.vi"("Device In"=w457, "Commands"=T9."Close_TL", "error in"=w453) -> ("error out"=w452:errorcluster)  [unwired: 9 in, 3 out]
                                n351 = call "TL_ALL_on_v2.vi"("error in"=w452) -> ()  [unwired: 11 in]
                                n352 = Wait (ms)(milliseconds to wait=u32 5000) -> ()  [unwired: 1 out]
                                }
                                }
                                }
                              }
                            }
                          }
                          n353 = Or(x=w390, y="Cancel Offline") -> (x .or. y?=w389:bool)
                        }
                      }
                    }
                  }
                  frame #1 {
                    # "CODE REMOVED!!!"
                    # "Reading the output power of the laser transmitter from the Ophir power meter, once read, convert to corresponding pulse energy and plot"
                  }
                  frame #2 {
                    # "Added in the ability to interactively control the ThorLab  setting (just etalon temp for now)"
                    # "CODE REMOVED!!!"
                    # "Wait 'Scalar Wait Time' for buffers to clear of online contiminated offline data"
                    n354 = event shown="[0] Timeout" {
                      selector: _ -> [_ _ _ _]
                      dyn-events: _ -> [_ _ _ _]
                      timeout: 1 -> [_ _ _ _]
                      event Timeout {
                        n355 = event-data() -> ()  [unwired: 1 in, 2 out]
                      }
                      event "Settings.EtalonTEC": Value Change {
                        # "Generating a command string\nto update the etalon"
                        n356 = event-data() -> ()  [unwired: 1 in, 5 out]
                        n357 = local read "Settings"() -> (w463:T6)
                        n358 = Unbundle By Name(w463) -> ("EtalonTEC"=w462:dbl)
                        n359 = Bundle By Name(cluster=w463, "EtalonTEC"=w462, "Module"=T11."Etalon TEC") -> (w465:T6)
                        n360 = call "TL_Driver.vi"("Device In"=refnum<visa-resource-name> "ThorLabs", "Commands"=T9."SET", "Settings"=w465) -> ("Readings"=w464:T5)  [unwired: 9 in, 3 out]
                        n361 = local write "Settings"(w465) -> ()
                        n362 = local write "Readings"(w464) -> ()
                      }
                      event "Settings.OnLineLD": Value Change {
                        # "Generating a command string\nto update the Online LD"
                        n363 = event-data() -> ()  [unwired: 1 in, 5 out]
                        n364 = local read "Settings"() -> (w470:T6)
                        n365 = Unbundle By Name(w470) -> ("OnLineLD"=w469:dbl)
                        n366 = Bundle By Name(cluster=w470, "OnLineLD"=w469, "Module"=T11."On Line LD") -> (w472:T6)
                        n367 = call "TL_Driver.vi"("Device In"=refnum<visa-resource-name> "ThorLabs", "Commands"=T9."SET", "Settings"=w472) -> ("Readings"=w471:T5)  [unwired: 9 in, 3 out]
                        n368 = local write "Settings"(w472) -> ()
                        n369 = local write "Readings"(w471) -> ()
                      }
                      event "Settings.OffLineLD": Value Change {
                        # "Generating a command string\nto update the Offline LD"
                        n370 = event-data() -> ()  [unwired: 1 in, 5 out]
                        n371 = local read "Settings"() -> (w477:T6)
                        n372 = Unbundle By Name(w477) -> ("OffLineLD"=w476:dbl)
                        n373 = Bundle By Name(cluster=w477, "OffLineLD"=w476, "Module"=T11."Off Line LD") -> (w479:T6)
                        n374 = call "TL_Driver.vi"("Device In"=refnum<visa-resource-name> "ThorLabs", "Commands"=T9."SET", "Settings"=w479) -> ("Readings"=w478:T5)  [unwired: 9 in, 3 out]
                        n375 = local write "Settings"(w479) -> ()
                        n376 = local write "Readings"(w478) -> ()
                      }
                    }
                  }
                  frame #3 {
                    w513 = 1 ("dimension size")
                    w516 = 1
                    # "Plotting the normalized relative \nbackscatter"
                    # "Calculating the normalized relative backscatter"
                    # "Calculating/Plotting smoothed data,\ncross sections etc."
                    # "Pick off data with\nout header"
                    # "Calculate mean bin by bin mean"
                    # "Reading in 'Integration Period (Seconds)' of data"
                    # "Read the offline data from the scalar card, perform smoothing, calculate normalized relative backscatter, and plot"
                    # "File path in MATLAB script is of old dial is:\nF:\\Micropulse DIAL\\Micropulse DIAL Matlab\\\nFinal Overlap Function.mat')];"
                    # "Collects Data From Card,\nSends It To The Chart,\nAnd Saves A Copy As A\nFile If Option Selected On\nFront Panel"
                    n377 = for {
                      N: "Data Reads (number of loops)" -> [_]
                      tunnel: [w549] -> w546 mode=indexing
                      tunnel: [w548] -> w528 mode=indexing
                      # "Read in latest scalar card data from \n'Scalar Data' global variable that \nscaler.vi is writing to, then wait 1 sec\nfor next batch of data"
                      n378 = global read "AMCS_Data.vi" "AMCS_Data"() -> (w550:u16[][])
                      n379 = disable-structure shown="Disabled" {
                        frame Disabled {
                          n380 = global read "Scalar_Data.vi" "Scalar Data  2"() -> ()  [unwired: 1 out]
                          n381 = global read "Scalar_Data.vi" "Scalar Data  4"() -> ()  [unwired: 1 out]
                        }
                        frame Enabled {
                        }
                      }
                      n382 = Index Array(array=w550, index (row) #1=1 ("index (row)"), index (row) #2=3 ("index (row)")) -> (element #1=w549:u16[], element #2=w548:u16[])  [unwired: 2 in]
                    }
                    n383 = local read "Total DIAL Integration Time (Minutes)"() -> (w537:i32)
                    n384 = Divide(x=w537, y="Data Reads (number of loops)") -> (x/y=w535:dbl)
                    n385 = local read "Total Aerosol Integration Time (Minutes)"() -> (w539:dbl)
                    n386 = Multiply(x=w535, y=60.0) -> (x*y=w521:dbl)
                    n387 = local read "background length"() -> (w485:i32)
                    n388 = local read "background start"() -> (w486:u32)
                    n389 = Transpose 2D Array(2D array=w546) -> (transposed array=w545:u16[][])
                    n390 = Transpose 2D Array(2D array=w528) -> (transposed array=w527:u16[][])
                    n391 = Divide(x=w539, y="Data Reads (number of loops)") -> (x/y=w540:dbl)
                    n392 = for {
                      tunnel: w545 -> [w556] mode=indexing
                      tunnel: [w555] -> w547 mode=indexing
                      tunnel: w527 -> [w554] mode=indexing
                      tunnel: [w553] -> _ mode=indexing
                      tunnel: [w553] -> w524 mode=indexing
                      n393 = call-poly <vilib>:"Mean.vi"("X"=w556) -> ("mean"=w555:dbl)  [unwired: 1 out]
                      n394 = call-poly <vilib>:"Mean.vi"("X"=w554) -> ("mean"=w553:dbl)  [unwired: 1 out]
                    }
                    n395 = local read "bins"() -> (w514:u32)
                    n396 = Multiply(x=w540, y=60.0) -> (x*y=w504:dbl)
                    n397 = Array Subset(array=w524, index=w513, length=w514) -> (w525:dbl[])
                    "Off-Line Bin Readings 2" <- w525
                    n398 = Array Subset(array=w547, index=w513, length=w514) -> (w523:dbl[])
                    "Off-Line  Bin Readings" <- w523
                    n399 = Array Subset(array=w525, index=w486, length=w485) -> (w526:dbl[])
                    n400 = Array Subset(array=w523, index=w486, length=w485) -> (w544:dbl[])
                    n401 = local read "Smoothed Bins"() -> (w482:dbl)
                    n402 = call-poly <vilib>:"Mean.vi"("X"=w526) -> ("mean"=w492:dbl)  [unwired: 1 out]
                    n403 = call-poly <vilib>:"Mean.vi"("X"=w544) -> ("mean"=w493:dbl)  [unwired: 1 out]
                    n404 = local read "Index"() -> (w503:i32)
                    n405 = Subtract(x=w525, y=w492) -> (x-y=w505:dbl[])
                    n406 = Subtract(x=w523, y=w493) -> (x-y=w519:dbl[])
                    n407 = call "Ring Buffer Offline Far.vi"("Index"=w503, "Profiles to Average"=w521, "Input Array"=w519) -> ("AvgArray"=w542:dbl[], "RingBufferOut"=→"RingBuffer offline far":dbl[][])  [unwired: 7 in]
                    n408 = call "Ring Buffer Aerosol Far.vi"("Index"=w503, "Profiles to Average"=w504, "Input Array"=w519) -> ("AvgArray"=w538:dbl[], "RingBufferOut"=→"RingBuffer aerosol far":dbl[][])  [unwired: 7 in]
                    n409 = call "Ring Buffer Offline Near.vi"("Index"=w503, "Profiles to Average"=w521, "Input Array"=w505) -> ("AvgArray"=w522:dbl[], "RingBufferOut"=→"RingBuffer offline near":dbl[][])  [unwired: 7 in]
                    n410 = call "Ring Buffer Aerosol Near.vi"("Index"=w503, "Profiles to Average"=w504, "Input Array"=w505) -> ("AvgArray"=w501:dbl[], "RingBufferOut"=→"RingBuffer aerosol near":dbl[][])  [unwired: 7 in]
                    n411 = Reshape Array(w519, w513, w514) -> (→"raw counts":dbl[][])
                    n412 = Reshape Array(w505, w513, w514) -> (→"raw counts near":dbl[][])
                    n413 = call "Smooth Arrray.vi"("smooth size"=w482, "Raw Array"=w542) -> ("Smoothed Array"=→"Off-Line Smoothed":dbl[])  [unwired: 9 in]
                    n414 = call "Smooth Arrray.vi"("smooth size"=w482, "Raw Array"=w538) -> ("Smoothed Array"=w512:dbl[])  [unwired: 9 in]
                    "Aerosol Smoothed" <- w512
                    n415 = call "Smooth Arrray.vi"("smooth size"=w482, "Raw Array"=w522) -> ("Smoothed Array"=→"Off-Line Smoothed 2":dbl[])  [unwired: 9 in]
                    n416 = call "Smooth Arrray.vi"("smooth size"=w482, "Raw Array"=w501) -> ("Smoothed Array"=w484:dbl[])  [unwired: 9 in]
                    "Aerosol Smoothed 2" <- w484
                    n417 = local read "Number of Accumulates"() -> (w488:u32)
                    n418 = local read "Temperature (C)"() -> (w534:dbl)
                    n419 = local read "Pressure (mb)"() -> (w533:dbl)
                    n420 = script code="%accum_num=10000;     % scaler card setting number of accumulations\nt_bin = 500e-9                 % scaler card setting time per bin\n%t_d = 37.3e-9;                % APD dead time from spec sheet\n\n% conversion from accumulated counts to count rate  (c/s)\nc_convert = 1./t_bin./accum_num;\nCR_far = p_raw_far.*c_convert;\nCR_near = p_raw_near.*c_convert;\nCR_total_far = (p_raw_far+b_far).*c_convert;\nCR_total_near = (p_raw_near+b_near).*c_convert;\nb_CR_far =b_far.*c_convert;\nb_CR_near =b_near.*c_convert;\n\n% create a range array\nsize_p =  size(p_raw_far,2);\nr = (75:75:size_p*75)./1e3; \n    \n%APD correction factor\n D_far = 1./(1-(t_d*CR_total_far));\n D_near = 1./(1-(t_d*CR_total_near));\n\n %Calculating normalize relative backscatter profile\n nrb_far = CR_far.*D_far.*r.^2.*1e-6;\n nrb_near = CR_near.*D_near.*r.^2.*1e-6;"("E"=6.0 ("Real"), "temp"=w534, "press"=w533, "p_raw_far"=w512, "b_far"=w493, "b_near"=w492, "p_raw_near"=w484, "accum_num"=w488, "t_d"="dead time") -> ("nrb_far"=w507:cdb[], "D_far"=w498:dbl[], "nrb_near"=w506:cdb[], "D_near"=w497:dbl[], "b_CR_far"=w490:dbl, "b_CR_near"=w489:dbl)  [unwired: 1 in, 1 out]
                    n421 = local read "bins"() -> (w515:u32)
                    n422 = local read "Altitude Array (km)"() -> (w509:dbl[])
                    n423 = Bundle(w490, w489) -> (→"?":cluster{dbl, dbl})  [unwired: 1 in]
                    n424 = Build Array(w507, w506) -> (w511:cdb[][])
                    n425 = Build Array(w498, w497) -> (w496:dbl[][])
                    n426 = Reshape Array(w506, w516, w515) -> (→"NRB 2":cdb[][])
                    n427 = Reshape Array(w507, w516, w515) -> (→"NRB":cdb[][])
                    n428 = Build Array(w509, w509) -> (w508:dbl[][])
                    n429 = call "Convert to Dynamic Data7"("2D Array"=w496) -> ("Dynamic Data Type"=w495:dynamicdata)  [unwired: 3 in]
                    n430 = call "Convert to Dynamic Data3"("2D Array"=w511) -> ("Dynamic Data Type"=w510:dynamicdata)  [unwired: 3 in]
                    n431 = call "Convert to Dynamic Data4"("2D Array"=w508) -> ("Dynamic Data Type"=w499:dynamicdata)  [unwired: 3 in]
                    n432 = call "Build XY Graph2"("Y Input"=w499, "X Input"=w510) -> ("XY Graph"=→"NRB plot":cluster{"Y":dbl[], "Y":dbl[]}[])  [unwired: 3 in, 6 out]
                    n433 = call "Build XY Graph4"("Y Input"=w499, "X Input"=w495) -> ("XY Graph"=→"Correction":cluster{"Y":dbl[], "Y":dbl[]}[])  [unwired: 3 in, 6 out]
                  }
                  frame #4 {
                    # "CODE REMOVED!!!"
                    # "Toggle Agiltron switch to online DBR"
                  }
                  frame #5 {
                    # "If 'Save Data?' is true, save all relavant offline info"
                    n434 = local read "Save Data?"() -> (w557:bool)
                    n435 = case shown="True" w557 {
                      frame False {
                        # "'Save Data?' is false, do nothing"
                      }
                      frame True {
                        # "Write only one data file at this time"
                        # "Retrive Julian Date"
                        # "'Save Data?' is true, save offline data to the Data Disk"
                        n436 = local read "Readings"() -> (w559:T5)
                        n437 = local read "Off-Line Bin Readings 2"() -> (w578:dbl[])
                        n438 = local read "Lambda Off Read (nm)"() -> (w580:dbl)
                        n439 = local read "Off-Line  Bin Readings"() -> (w585:dbl[])
                        n440 = local read "Relative Humdity (%)"() -> (w584:dbl)
                        n441 = local read "Temperature (C)"() -> (w582:dbl)
                        n442 = Unbundle By Name(w559) -> ("OffLineLD"=w558:dbl)
                        n443 = local read "T_bench"() -> (w581:sgl)
                        n444 = local read "Pressure (mb)"() -> (w583:dbl)
                        n445 = call "Julian_Date_2.vi"() -> ("Julian Date"=w579:dbl)  [unwired: 11 in]
                        n446 = Build Array (concatenate)(w579, w580, w558, w581, w582, w583, w584, w585) -> (w564:dbl[])
                        n447 = Build Array (concatenate)(w579, w580, w558, w581, w582, w583, w584, w578) -> (w561:dbl[])
                        n448 = local read "FF_Off_Ref"() -> (w566:refnum<file>)
                        n449 = local read "NF_Off_Ref"() -> (w563:refnum<file>)
                        n450 = local read "FF_Off_Ptr"() -> (w565:i64)
                        n451 = local read "NF_Off_Ptr"() -> (w562:i64)
                        n452 = Set File Position(offset (in bytes) (0)=w565, refnum=w566) -> (refnum out=w577:refnum<file>, error out=w575:errorcluster)  [unwired: 2 in]
                        n453 = Set File Position(offset (in bytes) (0)=w562, refnum=w563) -> (refnum out=w573:refnum<file>, error out=w571:errorcluster)  [unwired: 2 in]
                        n454 = Write to Binary File(file (use dialog)=w577, data=w564, error in=w575, 5:FALSE ("prepend array or string size? (T)")) -> (refnum out=w576:refnum<file>, error out=w574:errorcluster)  [unwired: 2 in, 1 out]
                        n455 = Write to Binary File(file (use dialog)=w573, data=w561, error in=w571, 5:FALSE ("prepend array or string size? (T)")) -> (refnum out=w572:refnum<file>, error out=w570:errorcluster)  [unwired: 2 in, 1 out]
                        n456 = Get File Position(4:w574, 7:w576) -> (2:w567:i64)  [unwired: 2 out]
                        n457 = Get File Position(4:w570, 7:w572) -> (2:w560:i64)  [unwired: 2 out]
                        n458 = local write "FF_Off_Ptr"(w567) -> ()
                        n459 = local write "NF_Off_Ptr"(w560) -> ()
                      }
                    }
                  }
                }
              }
              frame #4 {
                n460 = First Call?() -> (First Call?: T/F=w588:bool)
                n461 = Or(x="calculate absorption cross sections", y=w588) -> (x .or. y?=w586:bool)
                n462 = case shown="True" w586 {
                  frame False {
                  }
                  frame True {
                    # "calculate absorption cross sections from HITRAN data base"
                    n463 = local read "Off-Line Smoothed"() -> (w589:dbl[])
                    n464 = local read "Lambda On Read (nm)"() -> (w592:dbl)
                    n465 = local read "Lambda Off Set (nm)"() -> (w595:dbl)
                    n466 = local read "Temperature (C)"() -> (w593:dbl)
                    n467 = local read "Pressure (mb)"() -> (w594:dbl)
                    n468 = script code="hitran = dlmread('C:\\H2O_DIAL\\LabVIEW-2012\\Micropulse DIAL Matlab\\815nm_841nm_HITRAN_2008.csv', ',',[1 1 1676 8]);\n%hitran = dlmread('C:\\H2O_DIAL\\LabVIEW-2012\\Micropulse DIAL Matlab\\824nm_841nm_H2O_Spectral_Calc.csv', ',',[1 1 1209 7]);\n\n%Range vector in meters\nrange = ([75:75:size(Online,2)*75]);\n\nif lambda< 828\nlambda=828.195;\nelse\nlambda=lambda;\nend;\n\n%%\n\n%Voigt profile calculation\nWNmin = 1/(828+4)*1e7;  % 832.0 nm converted to wavenumber\nWNmax = 1/(828-4)*1e7;  % 824.0 nm converted to wavenumber\n\n%Find lines from WNmin to WNmax to calculate voigt profile\nline_indices = hitran(1:size(hitran,1),1)>WNmin & hitran(1:size(hitran,1),1)<WNmax;\n\nline = double(hitran(line_indices, 1:size(hitran,2)));\n\n%Calculate temperature and pressure profile\nT0 = 273+25; % surface temperature\nT0 = 273+T0_C;\nT = T0-0.0065.*range; % set to match the sounding\n\n% pressure in atmospheres\nP0  = 0.83; % surface pressure\nP0  = P0_mb/1000*0.986; %pressure in mb converted to atm\nP = P0.*(T0./T).^-5.5;   % set this value to match sounding\n\nT00 = 296;              % HITRAN reference temperature [K]\nP00 = 1;                % HITRAN reference pressure [atm]\nnu0_0 = line(:,1);      % absorption line center wavenumber from HITRAN [cm^-1]\nS0 = line(:,2);         % initial linestrength from HITRAN [cm^-1/(mol*cm^-2)]   \ngammal0 = line(:,4);    % air-broadened halfwidth at T_ref and P_ref from HITRAN [cm^-1/atm]\ngamma_s = line(:,5);    % self-broadened halfwidth at T_ref and P_ref from HITRAN [cm^-1/atm]\nE = line(:,6);          % ground state transition energy from HITRAN [cm^-1]  \nalpha = line(:,7);      % linewidth temperature dependence factor from HITRAN\ndelta = line(:,8);      % pressure shift from HiTRAN [cm^-1 atm^-1]\n\nnu_on = 1/(lambda)*1e7;\nnu_off = 1/(lambda_off)*1e7;\n\nfor i = 1:size(Online,2); % calculate the absorption cross section at each range\n  \n    nu0 = nu0_0+delta.*(P(i)./P00); % unclear if it should be Pi/P00  \n    gammal = gammal0.*(P(i)./P00).*((T00./T(i)).^alpha);    %Calculate Lorentz lineweidth at P(i) and T(i)\n\n    const.m = 18.015E-3./6.022E23; % mass of a single water molecule\n    const.k_B = 1.3806488e-23; % (J/K)\n    const.c = 299792458; % (m/s) (exact)\n \n    gammad = (nu0).*((2.0.*const.k_B.*T(i).*log(2.0))./(const.m.*const.c^2)).^(0.5);  %Calculate HWHM Doppler linewidth at T(i)\n     \n    % term 1 in the Voigt profile\n    y = (gammal./gammad).*((log(2.0)).^(0.5));\n    \n    % term 2 in the Voigt profile\n    x_on = ((nu_on-nu0)./gammad).*(log(2.0)).^(0.5);\n    x_off = ((nu_off-nu0)./gammad).*(log(2.0)).^(0.5);\n    \n    %setting up Voigt convolution\n    t = (-(size(line,1))/2:1:size(line,1)/2-1); %set up the integration spectral step size\n    t = repmat(t',1,length(x_on))';\n    x_on = repmat(x_on,1,length(t));\n    x_off = repmat(x_off,1,length(t));\n    y = repmat(y,1,length(t));\n    f_on = (exp(-t.^2.0))./(y.^2.0+(x_on-t).^2.0);  % combined Voigt term 1 and 2\n    f_off = (exp(-t.^2.0))./(y.^2.0+(x_off-t).^2.0);\n    %Voigt integration over all of the lines at the on and offline locations\n    z_on = trapz(t(1,:),f_on,2);\n    z_off =  trapz(t(1,:),f_off,2);\n    integral_on = z_on;\n    integral_off = z_off;\n    %Calculate linestrength at temperature T\n    S = S0.*((T00./T(i)).^(1.5)).*exp(1.439.*E.*((1./T00)-(1./T(i))));\n \n    %Calculate the Voigt profile\n    K_on = (y(:,1)./pi).*integral_on;\n    K_off = (y(:,1)./pi).*integral_off;\n    \n    %Calculate the Voigt profile absorption cross section [cm^2]\n    sigmav_on = S.*(1./gammad).*(((log(2.0))./pi).^(0.5)).*K_on; %.*far_wing_on;\n    sigmav_off = S.*(1./gammad).*(((log(2.0))./pi).^(0.5)).*K_off; %.*far_wing_off;\n    \n    %Sum contributions from all of the surrounding lines\n    sigma_on_total(i) = sum(sigmav_on);\n    sigma_off_total(i) = sum(sigmav_off);\n    \nend;"("lambda"=w592, "lambda_off"=w595, "P0_mb"=w594, "T0_C"=w593, "Online"=w589) -> ("sigma_on_total"=→"sigma_on_total":dbl[], "sigma_off_total"=→"sigma_off_total":dbl[])  [unwired: 1 in, 1 out]
                  }
                }
              }
              frame #5 {
                w606 = 1
                # "normalization factor\nfrom 300 to 450m"
                # "OPTICAL DEPTH PLOT"
                # "new rainbow color bar display"
                # "Data Processing Far Channel"
                # "new rainbow color bar display"
                # "Calculating the range resolved water vapor number density and plotting"
                n469 = local read "sigma_off_total"() -> (w629:dbl[])
                n470 = local read "sigma_on_total"() -> (w626:dbl[])
                n471 = local read "On-Line  Smoothed"() -> (w604:dbl[])
                n472 = local read "Off-Line Smoothed"() -> (w603:dbl[])
                n473 = local read "Off-Line Smoothed 2"() -> (w627:dbl[])
                n474 = local read "On-Line Smoothed 2"() -> (w628:dbl[])
                n475 = script code="%Time averaging in seconds.  180 Seconds =3 minutes\ntemporal_average = 180;\n\n%Spatial averaging in bins.  2 bins = 150 meters\nspatial_average = 2;\n\n%Creating r and r+deltar vectors..this can also be acsomplished using the\n%diff command\np_oni = Online(:,1:size(Online,2)-1);\n\np_onii = Online(:,2:size(Online,2));\n\np_offi = Offline(:,1:size(Offline,2)-1);\n\np_offii = Offline(:,2:size(Offline,2));\n\nInside = (p_oni.*p_offii)./(p_onii.*p_offi);\n\ndel_cross = 1./(2.*(sigma_on_total(1:size(Online,2)-1)-sigma_off_total(1:size(Offline,2)-1)).*75*100);\n\ndel_cross(isinf(del_cross)) = 0;\n\n%Calculating Number density\nN = del_cross.*log(Inside);\n\n%Spatial smoothing of the profiles\nfilter1 = ones(1,2)./2;\n\nN_1 = N;\n\nN_1_avg = filter2(filter1,N_1);\n\nfilter1 = ones(1,10)./10;\n\nN_2 = N;\n\nN_2_avg = filter2(filter1,N_2);\n\nN_new = zeros(size(N,1),size(N,2));\n \n%Using different averaging windows for different altitudes \nN_avg=[N_1_avg(:,1:40)';N_2_avg(:,41:size(N,2))']';\n\n\nw = N_avg.*1e6.*18.015./6.022e23"("Online"=w628, "Offline"=w627, "sigma_on_total"=w626, "sigma_off_total"=w629) -> ("N_avg"=w630:cdb[], "w"=w639:cdb[])  [unwired: 1 in, 1 out]
                n476 = script code="%Time averaging in seconds.  180 Seconds = 3 minutes\ntemporal_average = 180;\n\n%Spatial averaging in bins.  2 bins = 150 meters\nspatial_average = 2;\n\n%Creating r and r+deltar vectors..this can also be acsomplished using the\n%diff command\np_oni = Online(:,1:size(Online,2)-1);\n\np_onii = Online(:,2:size(Online,2));\n\np_offi = Offline(:,1:size(Offline,2)-1);\n\np_offii = Offline(:,2:size(Offline,2));\n\nInside = (p_oni.*p_offii)./(p_onii.*p_offi);\n\ndel_cross = 1./(2.*(sigma_on_total(1:size(Online,2)-1)-sigma_off_total(1:size(Offline,2)-1)).*75*100);\n\ndel_cross(isinf(del_cross)) = 0;\n\n%Calculating Number density\nN = del_cross.*log(Inside);\n\n%Spatial smoothing of the profiles\nfilter1 = ones(1,2)./2;\n\nN_1 = N;\n\nN_1_avg = filter2(filter1,N_1);\n\nfilter1 = ones(1,10)./10;\n\nN_2 = N;\n\nN_2_avg = filter2(filter1,N_2);\n\nN_new = zeros(size(N,1),size(N,2));\n \n%Using different averaging windows for different altitudes \nN_avg=[N_1_avg(:,1:40)';N_2_avg(:,41:size(N,2))']';\n\n \nw = N_avg.*1e6.*18.015./6.022e23"("Online"=w604, "Offline"=w603, "sigma_on_total"=w626, "sigma_off_total"=w629) -> ("N_avg"=w635:cdb[], "w"=w636:cdb[])  [unwired: 1 in, 1 out]
                n477 = local read "Time Resolution Per Bin(ns)"() -> (w605:u32)
                n478 = local read "bins"() -> (w631:u32)
                n479 = local read "Altitude Array (km)"() -> (w601:dbl[])
                n480 = Build Array(w636, w639) -> (w642:cdb[][])
                n481 = To Double Precision Float(number=w605) -> (double precision float=w624:dbl)
                n482 = Reshape Array(w635, w606, w631) -> (w646:cdb[][])
                n483 = Reshape Array(w630, w606, w631) -> (w633:cdb[][])
                n484 = Multiply(x=0.15, y=w624) -> (x*y=w622:dbl)
                n485 = Build Array(w635, w630) -> (w640:cdb[][])
                n486 = Divide(x=300.0, y=w622) -> (x/y=w619:dbl)
                n487 = Divide(x=450.0, y=w622) -> (x/y=w618:dbl)
                n488 = Build Array(w601, w601) -> (w625:dbl[][])
                n489 = call "Convert to Dynamic Data5"("2D Array"=w642) -> ("Dynamic Data Type"=w641:dynamicdata)  [unwired: 3 in]
                n490 = call "Convert to Dynamic Data2"("2D Array"=w640) -> ("Dynamic Data Type"=w637:dynamicdata)  [unwired: 3 in]
                n491 = Divide(x=w646, y=1e+17) -> (x/y=→"Water Vapor Number Density":cdb[][])
                n492 = Divide(x=w633, y=1e+17) -> (x/y=→"Water Vapor Number Density 2":cdb[][])
                n493 = call "Convert to Dynamic Data6"("Array"=w601) -> ("Dynamic Data Type"=w602:dynamicdata)  [unwired: 3 in]
                n494 = To Long Integer(number=w619) -> (32bit integer=w617:i32)
                n495 = To Long Integer(number=w618) -> (32bit integer=w616:i32)
                n496 = call "Convert to Dynamic Data"("2D Array"=w625) -> ("Dynamic Data Type"=w638:dynamicdata)  [unwired: 3 in]
                n497 = call "Convert to Dynamic Data8"("2D Array"=w625) -> ("Dynamic Data Type"=w643:dynamicdata)  [unwired: 3 in]
                n498 = Decrement(x=w617) -> (x-1=w614:i32)
                n499 = Decrement(x=w616) -> (x-1=w615:i32)
                n500 = call "Build XY Graph"("Y Input"=w638, "X Input"=w637) -> ("XY Graph"=→"Water Vapor Number Density  2":cluster{"Y":dbl[], "Y":dbl[]}[])  [unwired: 3 in, 6 out]
                n501 = call "Build XY Graph3"("Y Input"=w643, "X Input"=w641) -> ("XY Graph"=→"Absolute Humidity":cluster{"Y":dbl[], "Y":dbl[]}[])  [unwired: 3 in, 6 out]
                n502 = Array Subset(array=w604, index=w614, length=w615) -> (w613:dbl[])
                n503 = Array Subset(array=w603, index=w614, length=w615) -> (w612:dbl[])
                n504 = call-poly <vilib>:"Mean.vi"("X"=w613) -> ("mean"=w611:dbl)  [unwired: 1 out]
                n505 = call-poly <vilib>:"Mean.vi"("X"=w612) -> ("mean"=w610:dbl)  [unwired: 1 out]
                n506 = Divide(x=w611, y=w610) -> (x/y=w609:dbl)
                n507 = Multiply(x=w603, y=w609) -> (x*y=w608:dbl[])
                n508 = Divide(x=w604, y=w608) -> (x/y=w607:dbl[])
                n509 = Natural Logarithm(1:w607) -> (0:w598:dbl[])
                n510 = Multiply(x=-1.0, y=w598) -> (x*y=w597:dbl[])
                n511 = call "Convert to Dynamic Data9"("Array"=w597) -> ("Dynamic Data Type"=w600:dynamicdata)  [unwired: 3 in]
                n512 = call "Build OD Plot"("Y Input"=w602, "X Input"=w600) -> ("XY Graph"=→"Optical Depth":cluster{"Y":dbl[], "Y":dbl[]}[])  [unwired: 3 in, 6 out]
              }
            }
          }
        }
        "L_Count" <- w99
      }
    }
  }
  n513 = case shown="True" w3 {
    frame False {
    }
    frame True {
      # "close data files"
      # "Close Bristol WM"
      n514 = local read "Ophir PM On/Off"() -> (w650:bool)
      n515 = local read "Bristol Out"() -> (w655:i32)
      n516 = local read "NF_Off_Ref"() -> (w651:refnum<file>)
      n517 = local read "NF_On_Ref"() -> (w652:refnum<file>)
      n518 = local read "FF_Off_Ref"() -> (w653:refnum<file>)
      n519 = local read "WS_On/Off"() -> (w649:bool)
      n520 = local read "FF_On_Ref"() -> (w654:refnum<file>)
      n521 = case shown="True" w649 {
        frame False {
        }
        frame True {
          n522 = local read "WS visa"() -> (w660:refnum<visa-resource-name>)
          n523 = local read "ID_out"() -> (w657:refnum<k5>)
          n524 = call "T_RH_P.vi"("VISA in"=w660, "WS_Commands"=enum16{"OpenWS", "ReadTRHP", "CloseWS"}."CloseWS") -> ()  [unwired: 11 in, 3 out]
          n525 = call "ADAM6018_2.1.vi"("ADAM6018_Command"=enum16{"Open_Adam", "Read_Adam", "Close_Adam"}."Close_Adam", "ID_in"=w657) -> ()  [unwired: 11 in, 3 out]
        }
      }
      n526 = case shown="True" w650 {
        frame False {
        }
        frame True {
          n527 = local read "OphirPM"() -> (w656:T7)
          n528 = call "OphirClose.vi"("OphirPM"=w656) -> ()  [unwired: 18 in, 1 out]
        }
      }
      n529 = dll-call lib="C:/H2O_DIAL/LabVIEW-2012/Bristol WM V2_31b/CLDevIFace.dll" fn="CLCloseDevice"("CommPort"=w655) -> ()  [unwired: 5 in, 2 out]
      n530 = Close File(refnum=w654) -> ()  [unwired: 1 in, 2 out]
      n531 = Close File(refnum=w653) -> ()  [unwired: 1 in, 2 out]
      n532 = Close File(refnum=w652) -> ()  [unwired: 1 in, 2 out]
      n533 = Close File(refnum=w651) -> ()  [unwired: 1 in, 2 out]
    }
  }
  "FileHour" <- -1 ("FileHour")
  "DataOpen" <- FALSE
